vi "Text control 2 v6.9.vi"() -> ()   [LabVIEW 2016]
panel:
  in  "Tab Control":enum32{"Main", "Other parameters"}(tab)
  in  "Plot sample extrema vs time":bool
  out "Line running":i32
  out "Total lines":i32
  out "Path":path=path "C:/users/rlp38/09Apr2009LTtesting/test2.txt"
  out "I vs Vg":cluster{"Y data in":dbl[], "X data in":dbl[]}[](graph)
  out "Is max":dbl format="%.2e"
  out "Id max":dbl format="%.2e"
  out "Ig max":dbl format="%.2e"
  out "Imax vs time":cluster{"Y data in":dbl[], "X data in":dbl[]}[](graph)
  out "Imin vs time":cluster{"Y data in":dbl[], "X data in":dbl[]}[](graph)
  out "I vs Vd":cluster{"Y data in":dbl[], "X data in":dbl[]}[](graph)
  in  "Script":string="#pulsedstressV d 0.03 20 0 0.5 0.0827 5\n#\n#itime m\n#gaterangemode a\n#drainrangemode a\n#pulsed on 0.05 0 0.02\n#transfer d -10 40 1 5 40 35\n#transfer d -10 40 1 5 40 35\n#transfer d -10 40 1 5 40 35\n#output d 0 40 20 0 40 1\n#\n#\n#sample 1 0.008 221 6 0.003\n#samplei 400e-6 200 6 0.002 0.1\n#vsu2pulse -10 4\n#\n#stressV 0.016 0.03 2e-4 0.1e-3 11\n#stressI 220e-7 0.08 15\n#transfer s -1 1 0.5 -0.005 0.005 0.005\n#output s 0 0 0 -0.008 0.008 0.002"
  out "Command running:":string
  out "Serial port data":string
  out "Elapsed Time":dbl caption="Elapsed Time (s)"
  in  "Time Units":u16(ring)=1 items=["Seconds", "Minutes", "Hours"]
  in  "Time Offset":dbl caption="Set Start Time (s)"
  in  "Reset":bool
  in  "Auto Reset":bool
  in  "integration time":u32(slide) max=2 step=1 scale=0.0..2.0
  out "Is on":dbl format="%.2e"
  out "Id on":dbl format="%.2e"
  out "Ig on":dbl format="%.2e"
  out "Ion vs time":cluster{"Y data in":dbl[], "X data in":dbl[]}[](graph)
  out "Ioff vs time":cluster{"Y data in":dbl[], "X data in":dbl[]}[](graph)
  out "Ig min":dbl format="%.2e"
  out "Id min":dbl format="%.2e"
  out "Is min":dbl format="%.2e"
  out "Is off":dbl format="%.2e"
  out "Id off":dbl format="%.2e"
  out "Ig off":dbl format="%.2e"
  in  "Integration time (long)":dbl=0.32 min=0.04 max=2.0 step=0.02 format="%.2f"
  in  "Integration time (short)":dbl=0.0019 min=8e-05 max=0.0019 step=8e-05 format="%^.0e"
  in  "Drain: Compliance":dbl=0.001 format="%.8f"
  in  "Gate: Compliance":dbl=0.001 format="%.8f"
  in  "Interrupt scan":bool
  in  "Interrupt program":bool
  in  "Plot output curve extrema vs time":bool
  in  "Plot transfer curve extrema vs time":bool
  out "I vs time (Bias Stress)":cluster{"Y data in":dbl[], "X data in":dbl[]}[](graph)
  in  "Sample I - Probe 4 (Disabled)":u32(ring)=3 items=["SMU1  ", "SMU2  ", "SMU3  ", "SMU4  ", "SMU5  ", "SMU6  "]
  in  "Sample I - Source/Common":u32(ring) items=["SMU1  ", "SMU2  ", "SMU3  ", "SMU4  ", "SMU5  ", "SMU6  "]
  in  "Sample I - Probe 3 (Disabled)":u32(ring)=2 items=["SMU1  ", "SMU2  ", "SMU3  ", "SMU4  ", "SMU5  ", "SMU6  "]
  in  "Sample I - Drain/Gate":u32(ring)=1 items=["SMU1  ", "SMU2  ", "SMU3  ", "SMU4  ", "SMU5  ", "SMU6  "]
  in  "Sample - Probe 4":u32(ring)=3 items=["SMU1  ", "SMU2  ", "SMU3  ", "SMU4  ", "SMU5  ", "SMU6  "]
  in  "Sample - Source/Common":u32(ring) items=["SMU1  ", "SMU2  ", "SMU3  ", "SMU4  ", "SMU5  ", "SMU6  "]
  in  "Sample - Gate":u32(ring)=2 items=["SMU1  ", "SMU2  ", "SMU3  ", "SMU4  ", "SMU5  ", "SMU6  "]
  in  "Sample - Drain":u32(ring)=1 items=["SMU1  ", "SMU2  ", "SMU3  ", "SMU4  ", "SMU5  ", "SMU6  "]
  in  "Gate Range\nmode":u16(ring) items=["Auto", "Limited", "Fixed"]
  in  "Gate Range":u8(slide)=3 max=11 scale=0.0..11.0
  in  "Source/Drain\nRange mode":u16(ring) items=["Auto", "Limited", "Fixed"]
  in  "Source/Drain Range":u8(slide)=3 max=11 scale=0.0..11.0
  in  "Panel Controls":T1={"Emergency Stop"=refnum, "TransGraph Max"=1e-05, "Text/Graph (text=false)"=TRUE} {"TransGraph Max" format="%.2e"}
  in  "Panel Controls 2":T2={"Emergency Stop"=refnum, "TransGraph Max"=1e-05, "Text/Graph (text=false)"=TRUE, "TransGraph Min"=1e-11} {"TransGraph Min" format="%.2e"; "TransGraph Max" format="%.2e"}
  out "error out":errorcluster
  in  "Delay before read (ms)":u32=1000
  in  "byte count":u32=64
  in  "Serial End Mode for Reads":u16(ring)=2 items=["None", "LastBit", "TermChar"]
  in  "Timeout (ms)":u32=10000
  in  "Enable Termination\nChar (T)":bool=TRUE
  in  "Termination char\n(0xA = '\\n' = LF)\n(0xD = '\\r' = CR)":u8=13 format="%.0x"
  in  "flow control":u16(ring) items=["None"=0, "XON/XOFF"=1, "RTS/CTS"=2, "DTR/DSR"=4]
  in  "stop bits":u16(ring)=10 items=["1.0"=10, "1.5"=15, "2.0"=20]
  in  "parity":u16(ring) items=["None", "Odd", "Even", "Mark", "Space"]
  in  "data bits":u16=8 min=5 max=8 step=1
  in  "VISA resource name":refnum<visa-resource-name>="COM6"
  in  "baud rate":u32=9600
  out "Timings Indicator":T3
  in  "Timings (overwritten by the Front Panel)":T4={"integration time"=0, "Short/Long integration time"=0.00064, "hold time (sec)"=0.0, "delay time (sec)"=0.0, "Step Time (0 disables)"=0.0, "sweep method"=0, "Pulse period"=0.005, "Base voltage"=0.0, "Pulse width"=0.0005} {"Pulse width" min=0.0005 max=0.1 step=0.0001 format="%.4f"; "Base voltage" format="%^.4e"; "Pulse period" min=0.005 max=1.0 step=0.0001 format="%.4f"; "sweep method" items=["Continuous", "Pulsed"]; "Step Time (0 disables)" format="%.2f"; "delay time (sec)" format="%.4f"; "hold time (sec)" format="%.4f"; "Short/Long integration time" format="%^.0e"; "integration time" scale=0.0..2.0}
  in  "Probe 4":cluster{"on/off":bool, "Voltage":dbl} {"Voltage" min=-100.0 max=100.0 format="%.2f"}
  in  "Full Reset":bool
  in  "Standby":T5
  out "Probe 4 Indicator":cluster{"on/off":bool, "Voltage":dbl} {"Voltage" min=-100.0 max=100.0 format="%.2f"}
  in  "Transfer/Output - Drain":u32(ring)=1 items=["SMU1  ", "SMU2  ", "SMU3  ", "SMU4  ", "SMU5  ", "SMU6  "]
  in  "Transfer/Output - Gate":u32(ring)=2 items=["SMU1  ", "SMU2  ", "SMU3  ", "SMU4  ", "SMU5  ", "SMU6  "]
  in  "Transfer/Output - Source/Common":u32(ring) items=["SMU1  ", "SMU2  ", "SMU3  ", "SMU4  ", "SMU5  ", "SMU6  "]
  in  "Transfer/Output - Probe 4":u32(ring)=3 items=["SMU1  ", "SMU2  ", "SMU3  ", "SMU4  ", "SMU5  ", "SMU6  "]
  in  "Pulsed Stress V - Probe 4":u32(ring)=3 items=["SMU1  ", "SMU2  ", "SMU3  ", "SMU4  ", "SMU5  ", "SMU6  "]
  in  "Pulsed Stress V - Vextra":u32(ring)=1 items=["VSU1  ", "VSU2  "]
  in  "Pulsed Stress V - Drain":u32(ring)=1 items=["SMU1  ", "SMU2  ", "SMU3  ", "SMU4  ", "SMU5  ", "SMU6  "]
  in  "Pulsed Stress V - Source/Common":u32(ring) items=["SMU1  ", "SMU2  ", "SMU3  ", "SMU4  ", "SMU5  ", "SMU6  "]
  in  "Pulsed Stress V - Gate":u32(ring)=2 items=["SMU1  ", "SMU2  ", "SMU3  ", "SMU4  ", "SMU5  ", "SMU6  "]
  in  "FPP - Drain":u32(ring)=1 items=["SMU1  ", "SMU2  ", "SMU3  ", "SMU4  ", "SMU5  ", "SMU6  "]
  in  "FPP - Gate":u32(ring)=2 items=["SMU1  ", "SMU2  ", "SMU3  ", "SMU4  ", "SMU5  ", "SMU6  "]
  in  "FPP - Probe 1":u32(ring) items=["SMU1  ", "SMU2  ", "SMU3  ", "SMU4  ", "SMU5  ", "SMU6  "]
  in  "FPP - Probe 2":u32(ring)=3 items=["SMU1  ", "SMU2  ", "SMU3  ", "SMU4  ", "SMU5  ", "SMU6  "]
  in  "FPP - Source":u32(ring) items=["VSU1  ", "VSU2  "]
  in  "Stress V - Drain":u32(ring)=1 items=["SMU1  ", "SMU2  ", "SMU3  ", "SMU4  ", "SMU5  ", "SMU6  "]
  in  "Stress V - Gate":u32(ring)=2 items=["SMU1  ", "SMU2  ", "SMU3  ", "SMU4  ", "SMU5  ", "SMU6  "]
  in  "Stress V - Source/Common":u32(ring) items=["SMU1  ", "SMU2  ", "SMU3  ", "SMU4  ", "SMU5  ", "SMU6  "]
  in  "Stress I - Drain/Gate":u32(ring)=1 items=["SMU1  ", "SMU2  ", "SMU3  ", "SMU4  ", "SMU5  ", "SMU6  "]
  in  "Stress I - Source/Common":u32(ring) items=["SMU1  ", "SMU2  ", "SMU3  ", "SMU4  ", "SMU5  ", "SMU6  "]
  in  "VSU2 Stress - Source/Common":u32(ring) items=["SMU1  ", "SMU2  ", "SMU3  ", "SMU4  ", "SMU5  ", "SMU6  "]
  in  "VISA resource name in":refnum<visa-resource-name>="GPIB0::14::INSTR"
  in  "Gate":T6={"Gate Start"=0.0, "Gate Stop"=2.0, "Gate Step (linear only)"=1.0, "Gate Compliance"=0.0001, "Gate PComp"=0.0, "Range mode"=0, "Range"=6} {"Range" max=11 scale=0.0..11.0; "Range mode" items=["Auto", "Limited", "Fixed"]; "Gate PComp" format="%^.2e"; "Gate Compliance" format="%^.2e"; "Gate Step (linear only)" format="%^.4e"; "Gate Stop" format="%^.4e"; "Gate Start" format="%^.4e"}
  in  "Drain 2":T7={"Drain Start"=0.0, "Drain Stop"=2.0, "Drain Compliance"=0.0001, "Drain Step"=1.0, "Drain PComp"=0.0, "Range mode"=0, "Range"=6} {"Range" max=11 scale=0.0..11.0; "Range mode" items=["Auto", "Limited", "Fixed"]; "Drain PComp" format="%^.2e"; "Drain Step" format="%^.4e"; "Drain Compliance" format="%^.2e"; "Drain Stop" format="%^.4e"; "Drain Start" format="%^.4e"}
  # "Time"
  # "Syntax:\nitime [s|m|l] time(sec): [s|m|l] determines the integration time setting (small|medium|long) and time sets the value.\nNOTE: The value of the integration time has to be within the range allowed by its category (s|m|l), otherwise, the closest value will be used. (e.g. if the category is set to short but the time value is very long, the actual value used will be the maximum short integration time.\nIntegration times:\n    Short: Default: 640 us. Range: 8E-5 - 1.92E-3 seconds.\n    Medium: Fixed at 1 NPL cycle (0.02 seconds).\n    Long: Default: 16 NPL cycles (0.32 seconds). Range: 2-100 NPL cycles (0.04 seconds - 2 seconds).\ngaterangemode [a|l|f]\ndrainrangemode [a|l|f]\npulsed [on|off] PulsePeriod(sec) PulseBaseVoltage PulseONWidth(sec)\nstandby [on l off]\nwait NumMilliseconds\nwait-min NumMinutes\n# texthere = comment\nProbe4 [ON|OFF] Voltage\ntransfer [s|d] VgStart VgStop VgStep VdStart VdStop VdStep\noutput [s|d] VgStart VgStop VgStep VdStart VdStop VdStep\nsample Vg Vd NumSamples Time(s) SampleInterval(s)\nsamplei Idg NumSamples Time(s) SampleInterval(s) VDGcompliance\n100 samples is approximately 13 seconds with medium integration\n# if in doubt use SampleInterval(s) = 0.004\n    NOTE: When doing bias stress measurements, set the Time Units to \"Seconds\", as the \"sample\" command has been configured to give the output to seconds.\nstressV VG VD IGcompliance IDcompliance Duration(sec)\nstressI IDG VDGcompliance Duration(sec)\nvsu2pulse Bias Duration(s)\npulsedstressV [s|d] VEstop VgON VgOFF Period(s) PulseONwidth(s) Vd\nsample-fpp Vg Vd NumSamples Time\nresample-fpp Vg Vd\ntransfer-fpp [s|d] VgStart VgStop VgStep VdStart VdStop VdStep\noutput-fpp [s|d] VgStart VgStop VgStep VdStart VdStop VdStep\nserial SerialPortCommand"
  # "1\n2\n3\n4\n5\n6\n7\n8\n9\n10\n11\n12\n13\n14\n15\n16\n17\n18\n19\n20"
  # "SMUs"
  # "Serial port settings"
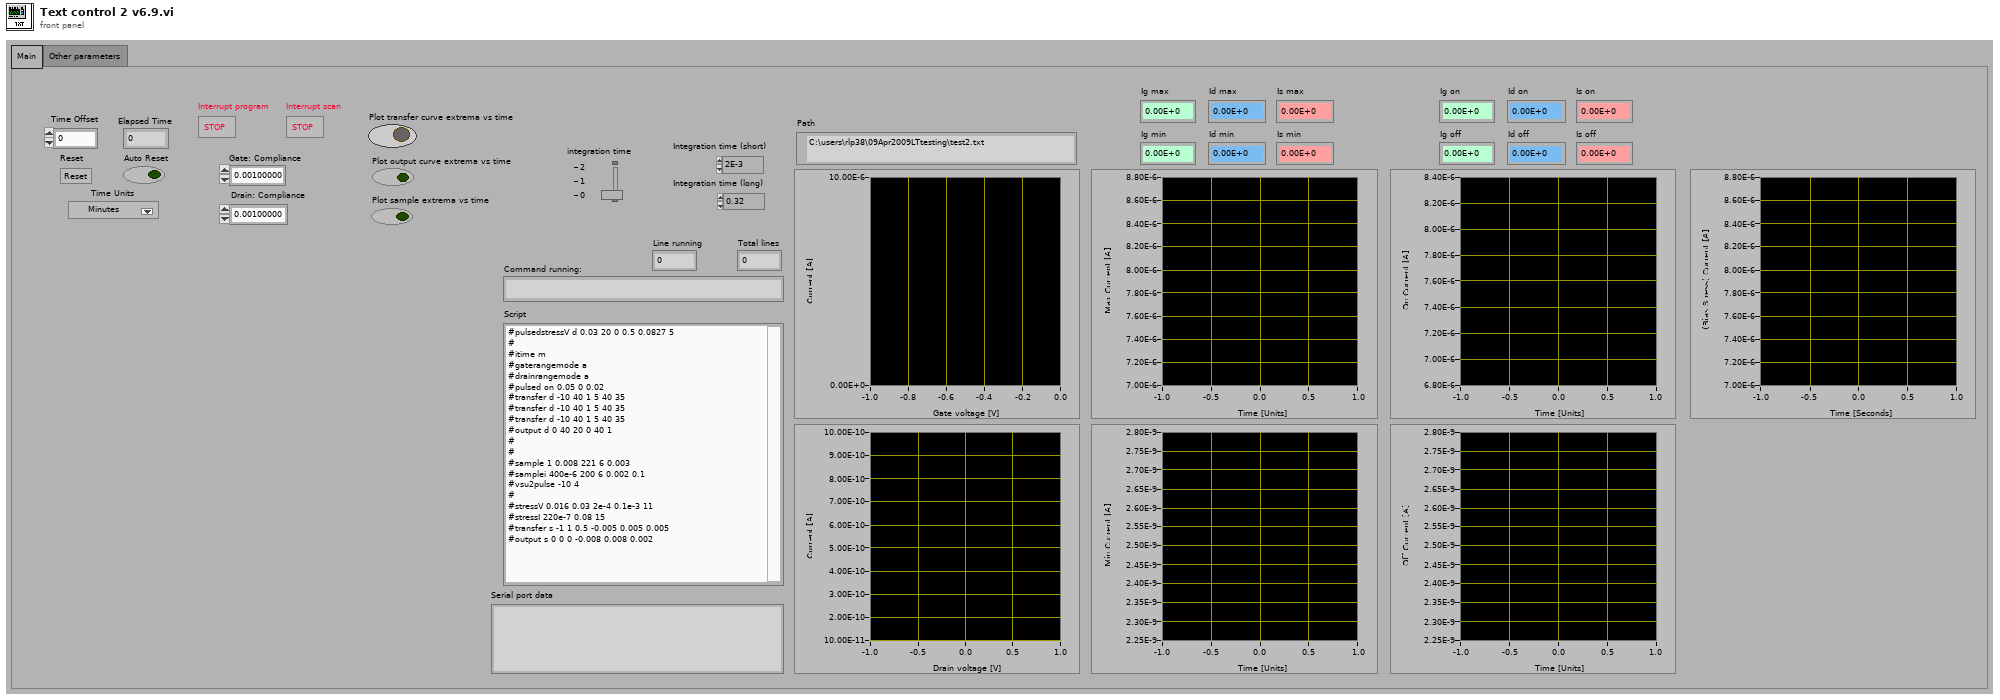
[diagram p1: front panel]
types:
  T1 = cluster{"Emergency Stop":refnum<vi>, "TransGraph Max":dbl, "Text/Graph (text=false)":bool}
  T2 = cluster{"Emergency Stop":refnum<vi>, "TransGraph Max":dbl, "Text/Graph (text=false)":bool, "TransGraph Min":dbl}
  T3 = cluster{"integration time (0:s, 1:m, 2:l)":u32, "Short/Long integration time":dbl, "hold time (sec)":dbl, "delay time (sec)":dbl, "Step Time (0 disables)":dbl, "sweep method":u16, "Pulse period":dbl, "Base voltage":dbl, "Pulse width":dbl}
  T4 = cluster{"integration time":u32, "Short/Long integration time":dbl, "hold time (sec)":dbl, "delay time (sec)":dbl, "Step Time (0 disables)":dbl, "sweep method":u16, "Pulse period":dbl, "Base voltage":dbl, "Pulse width":dbl}
  T5 = cluster{"Gate Standby":bool, "Drain Standby":bool}
  T6 = cluster{"Gate Start":dbl, "Gate Stop":dbl, "Gate Step (linear only)":dbl, "Gate Compliance":dbl, "Gate PComp":dbl, "Range mode":u16, "Range":u8}
  T7 = cluster{"Drain Start":dbl, "Drain Stop":dbl, "Drain Compliance":dbl, "Drain Step":dbl, "Drain PComp":dbl, "Range mode":u16, "Range":u8}
  T8 = enum16{"open", "replace", "create", "open or create", "replace or create", "replace or create with confirmation"}
  T9 = cluster{"V2 Start":dbl, "V2 Step":dbl, "Number of points":i32}
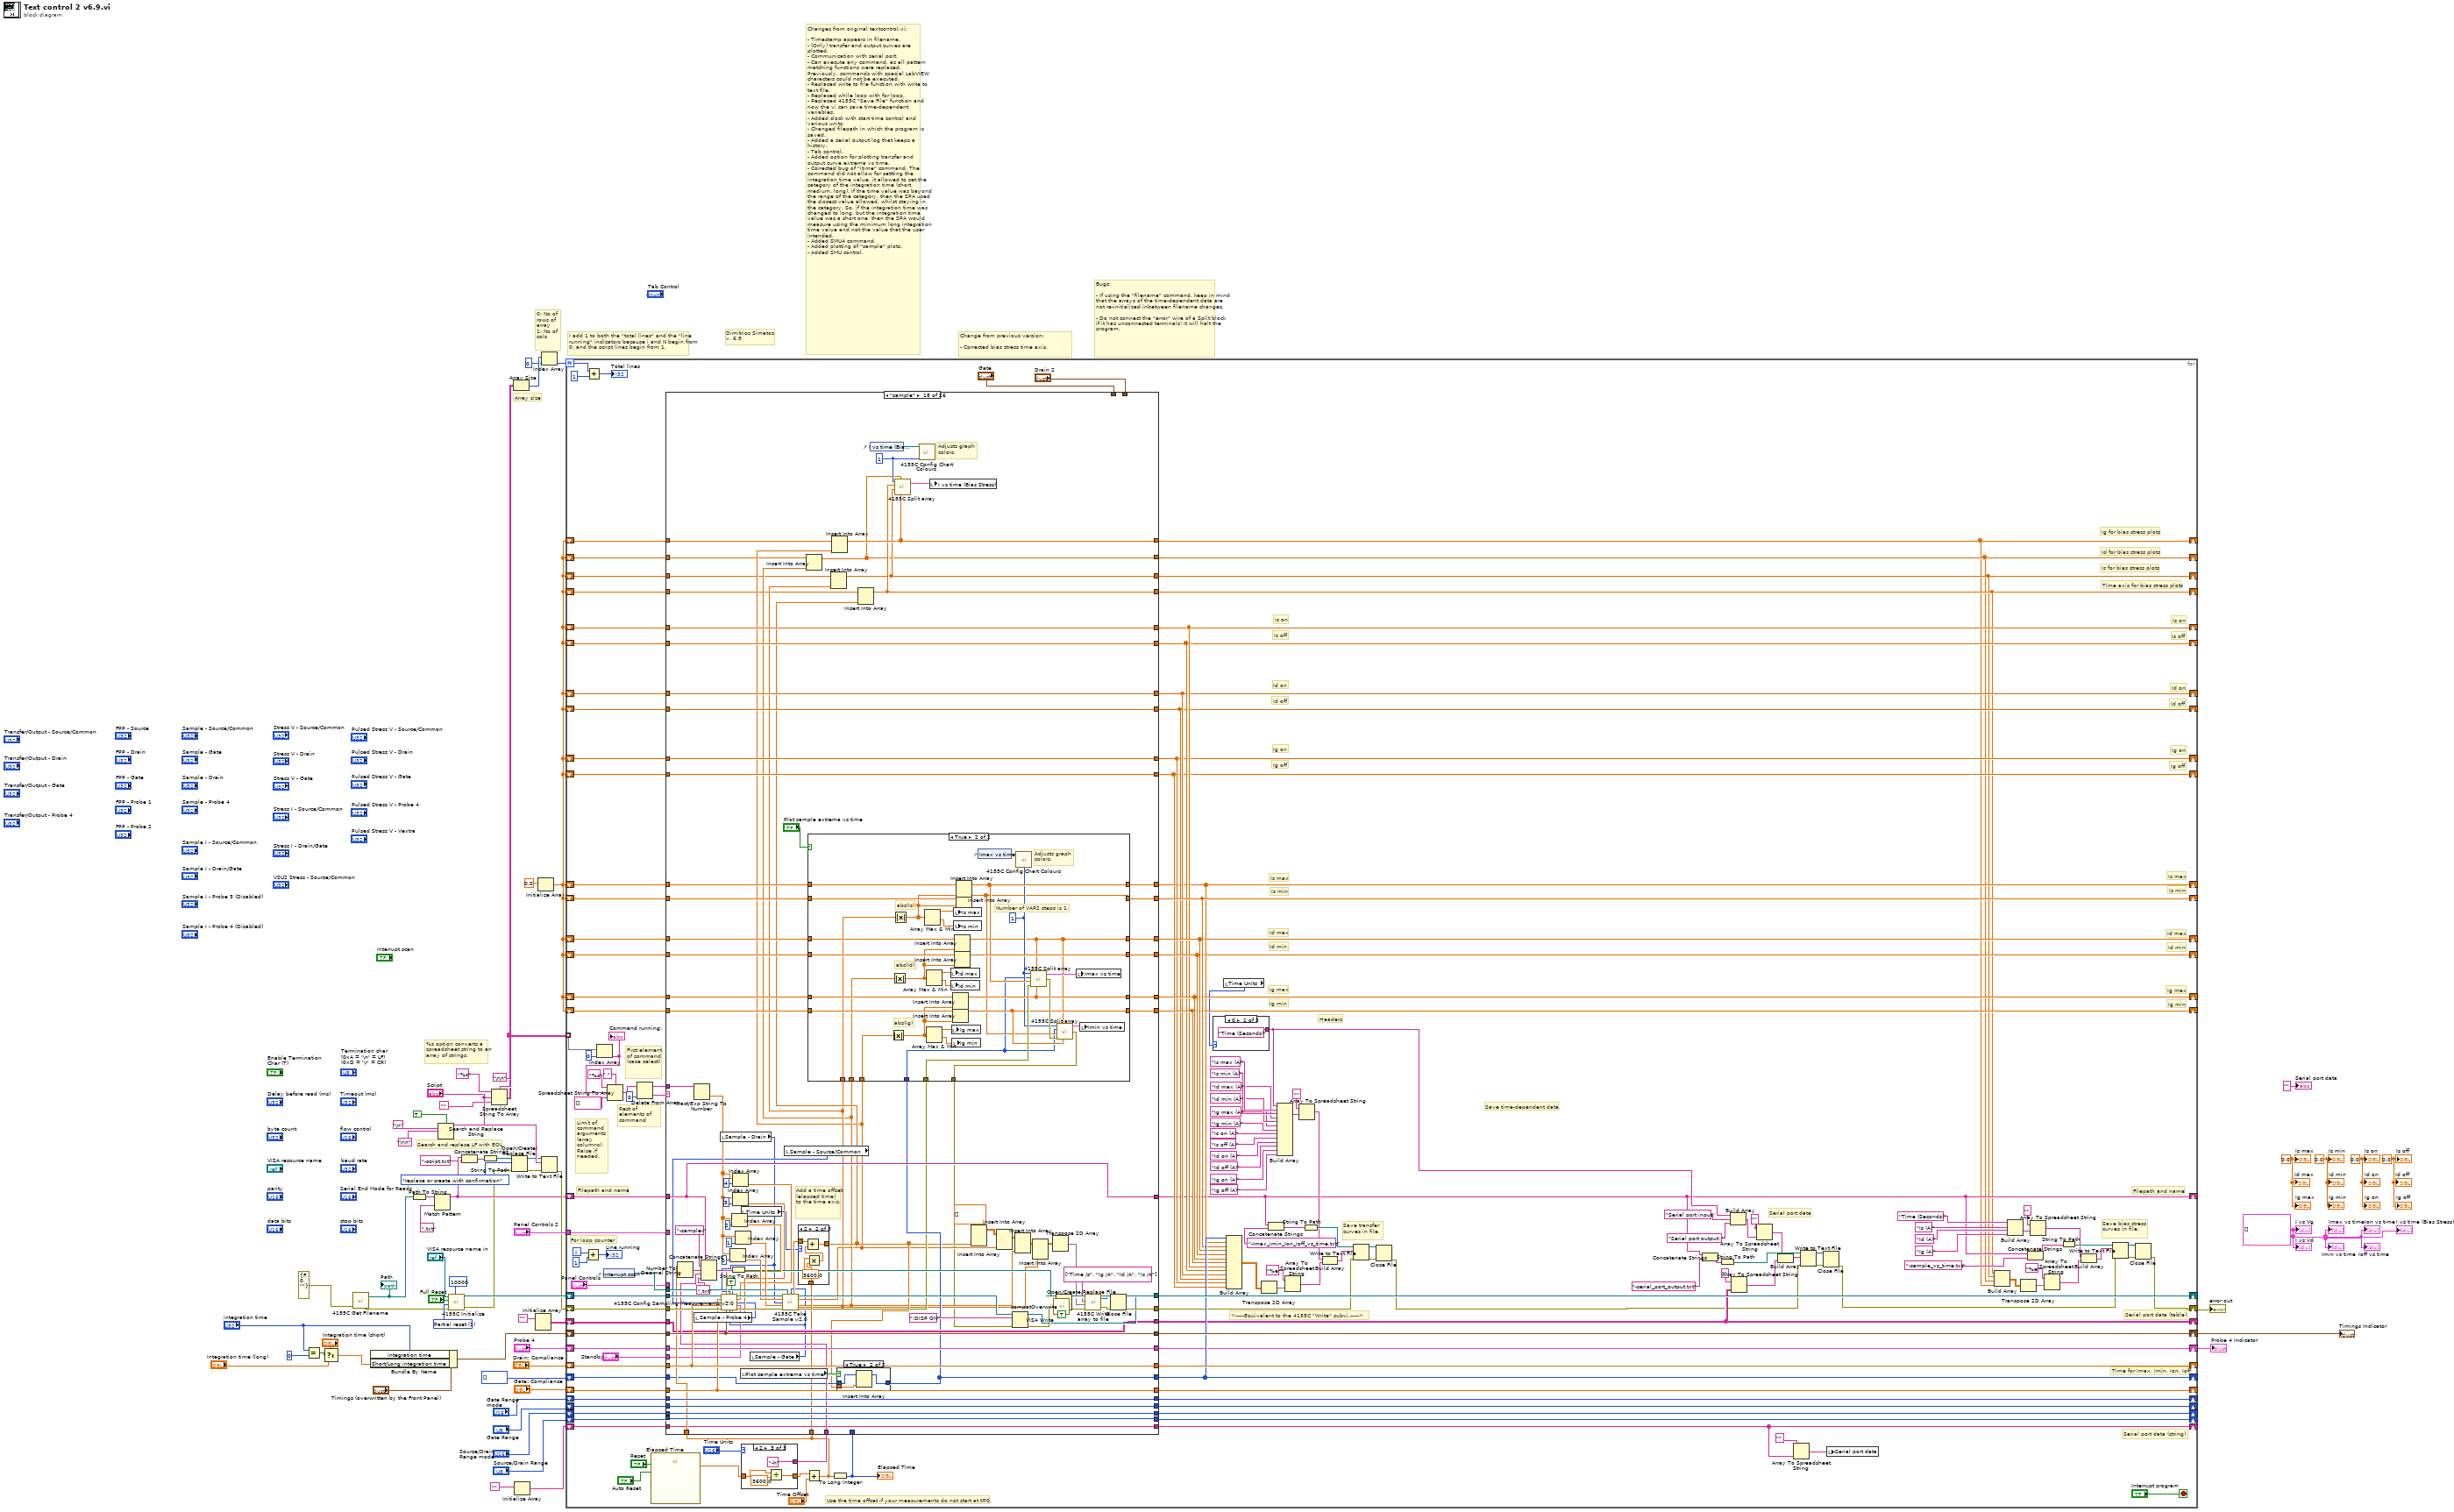
[diagram p0: block diagram]
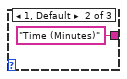
[diagram p2: hidden frame]
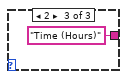
[diagram p3: hidden frame]
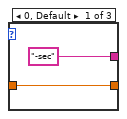
[diagram p4: hidden frame]
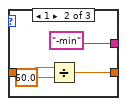
[diagram p5: hidden frame]
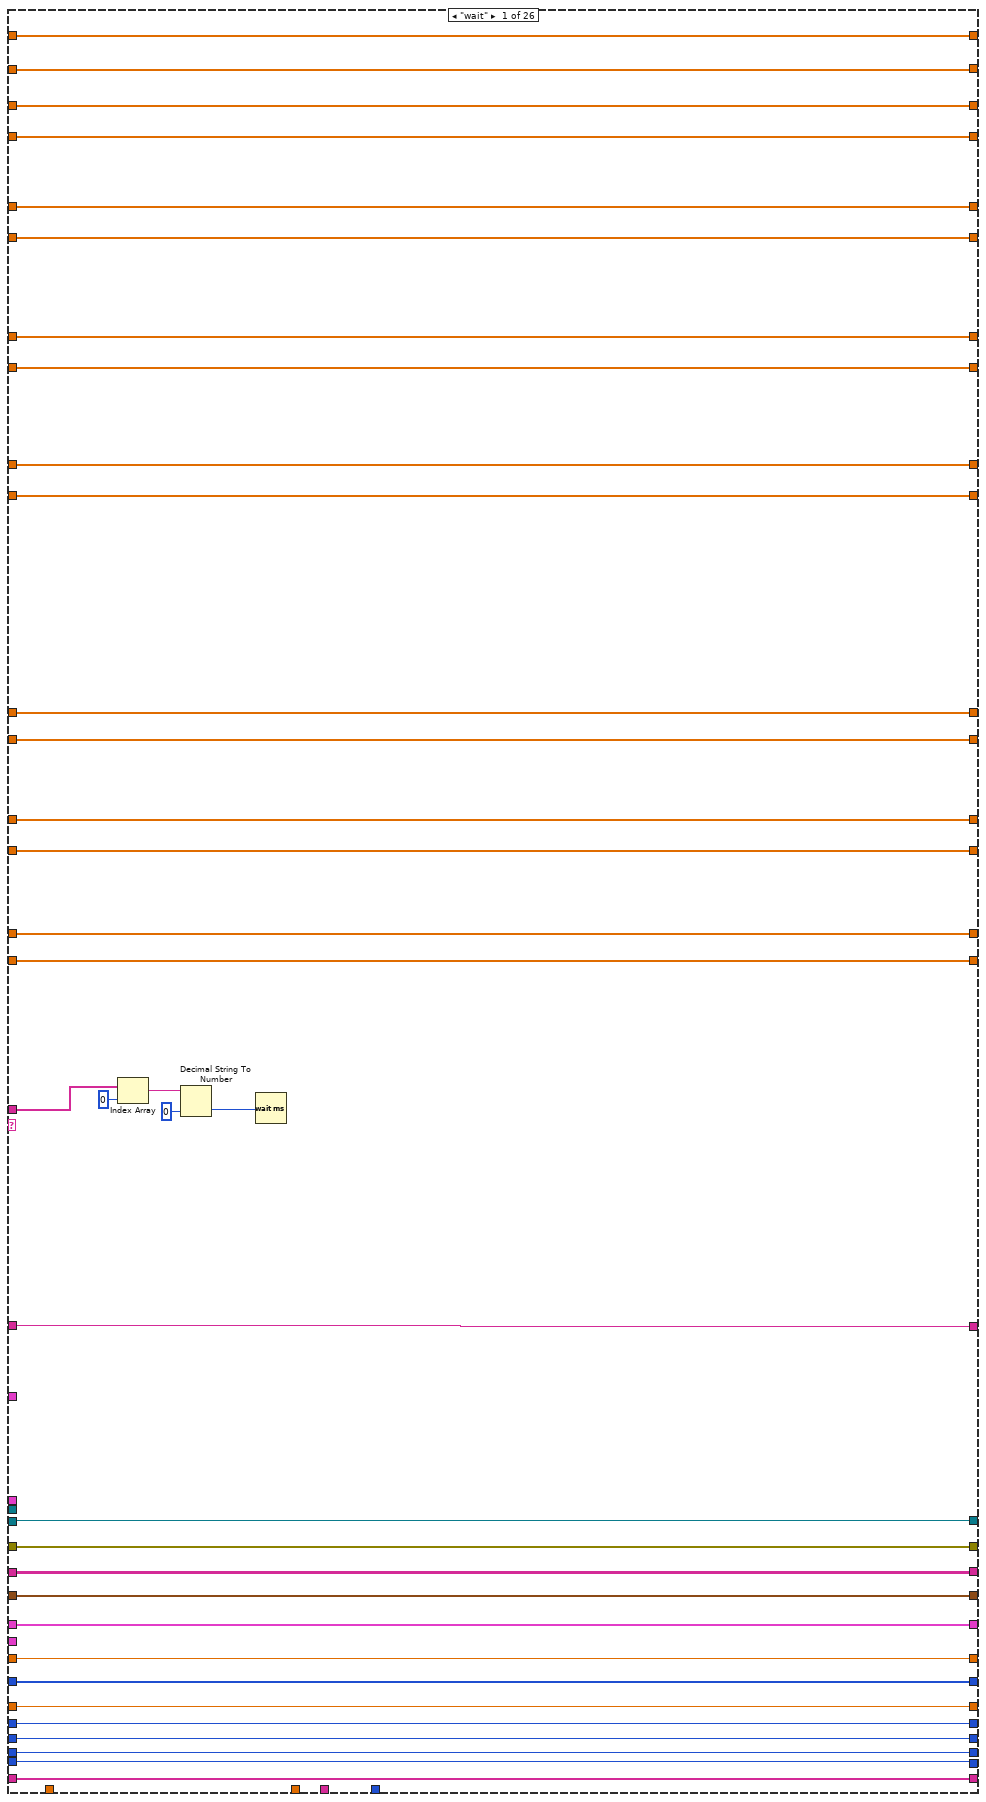
[diagram p6: hidden frame]
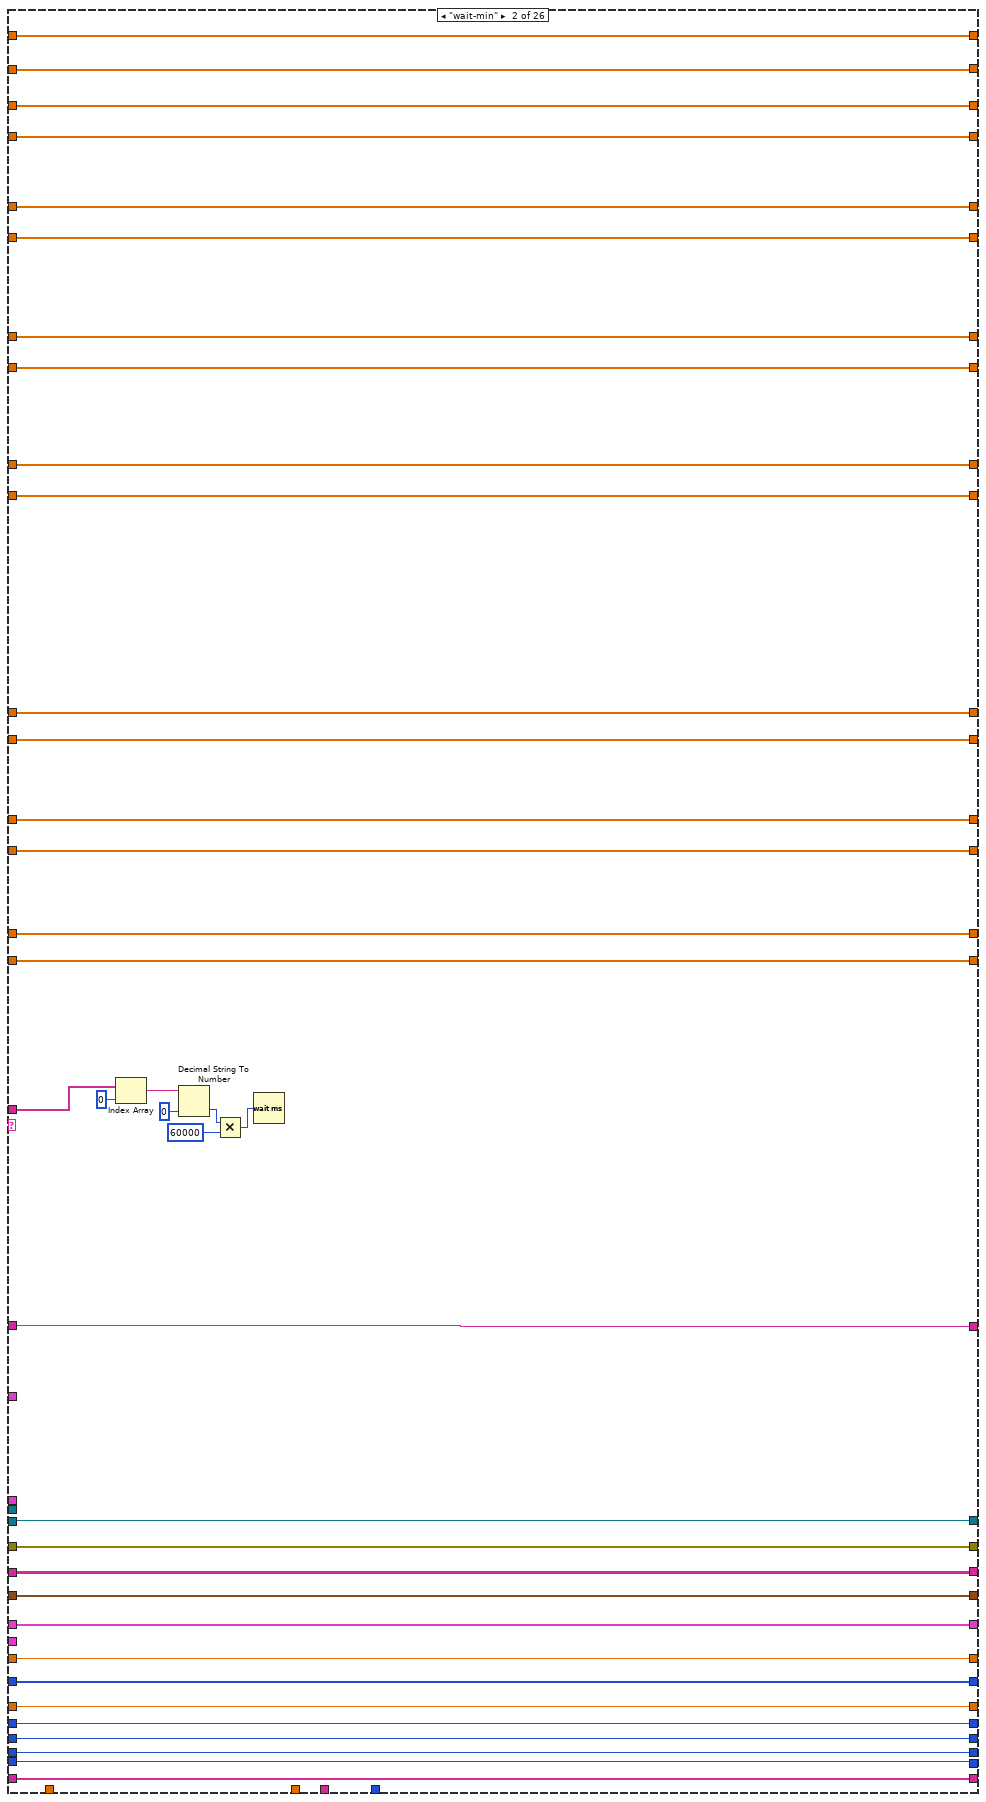
[diagram p7: hidden frame]
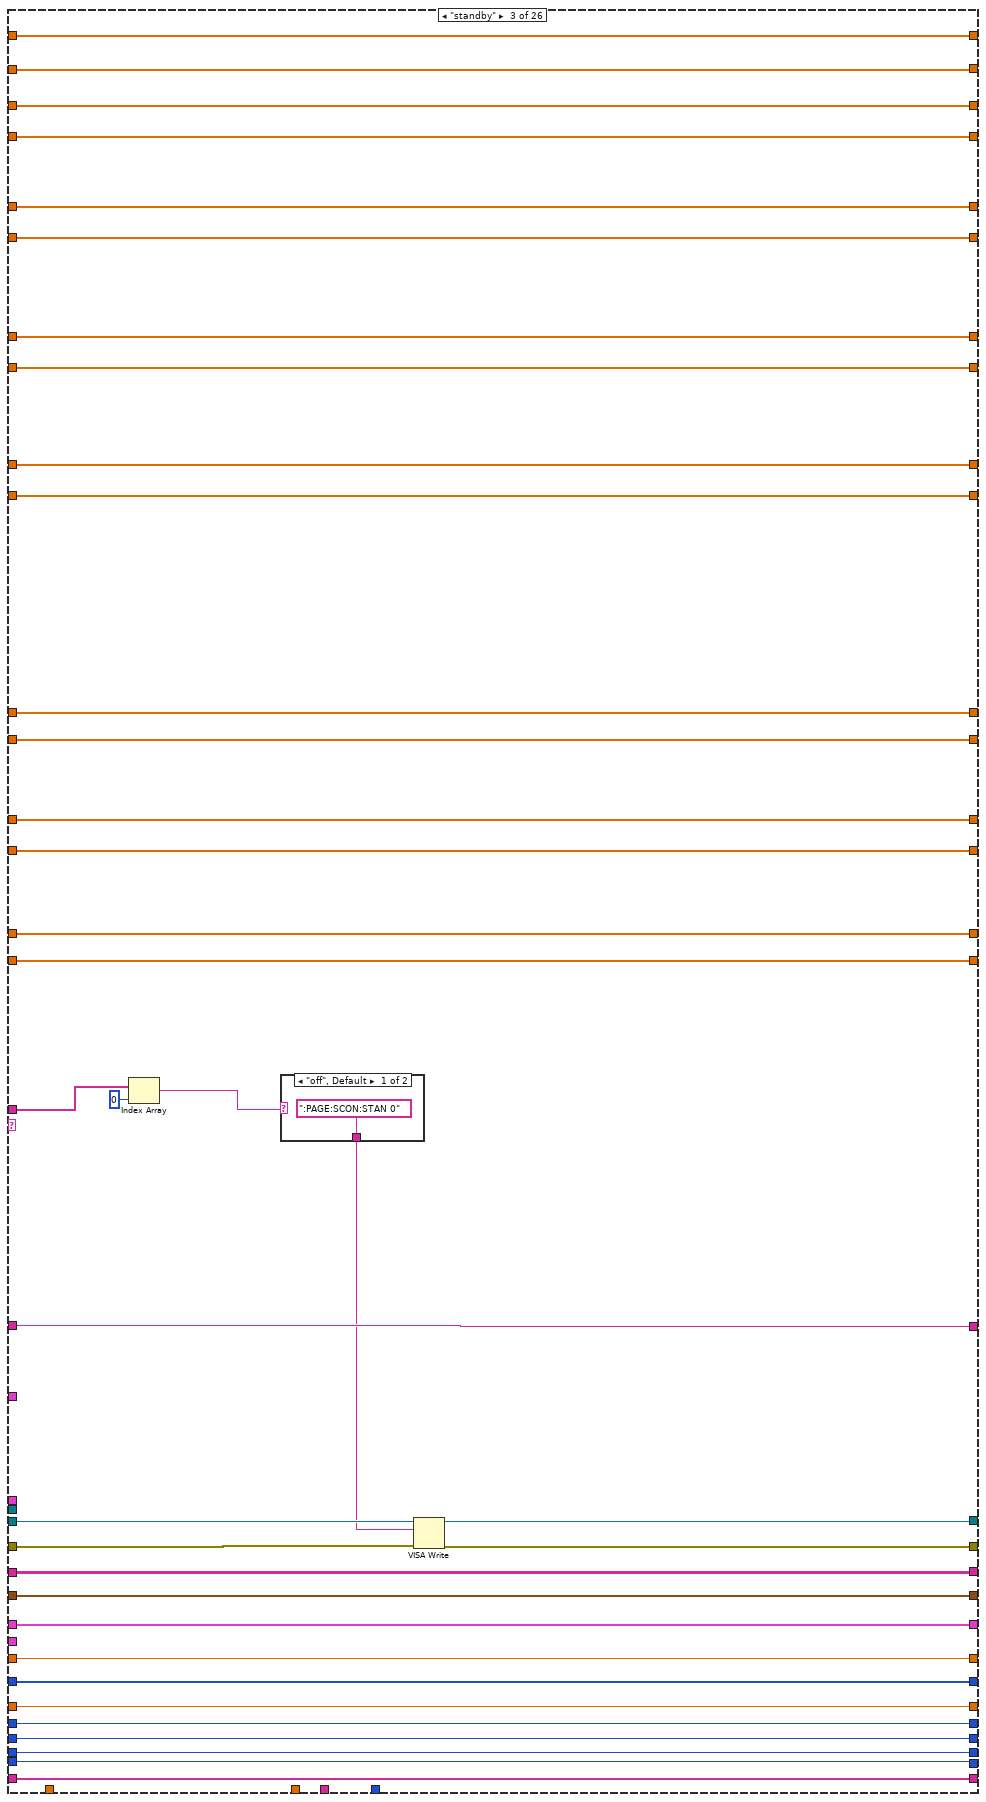
[diagram p8: hidden frame]
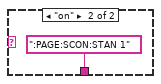
[diagram p9: hidden frame]
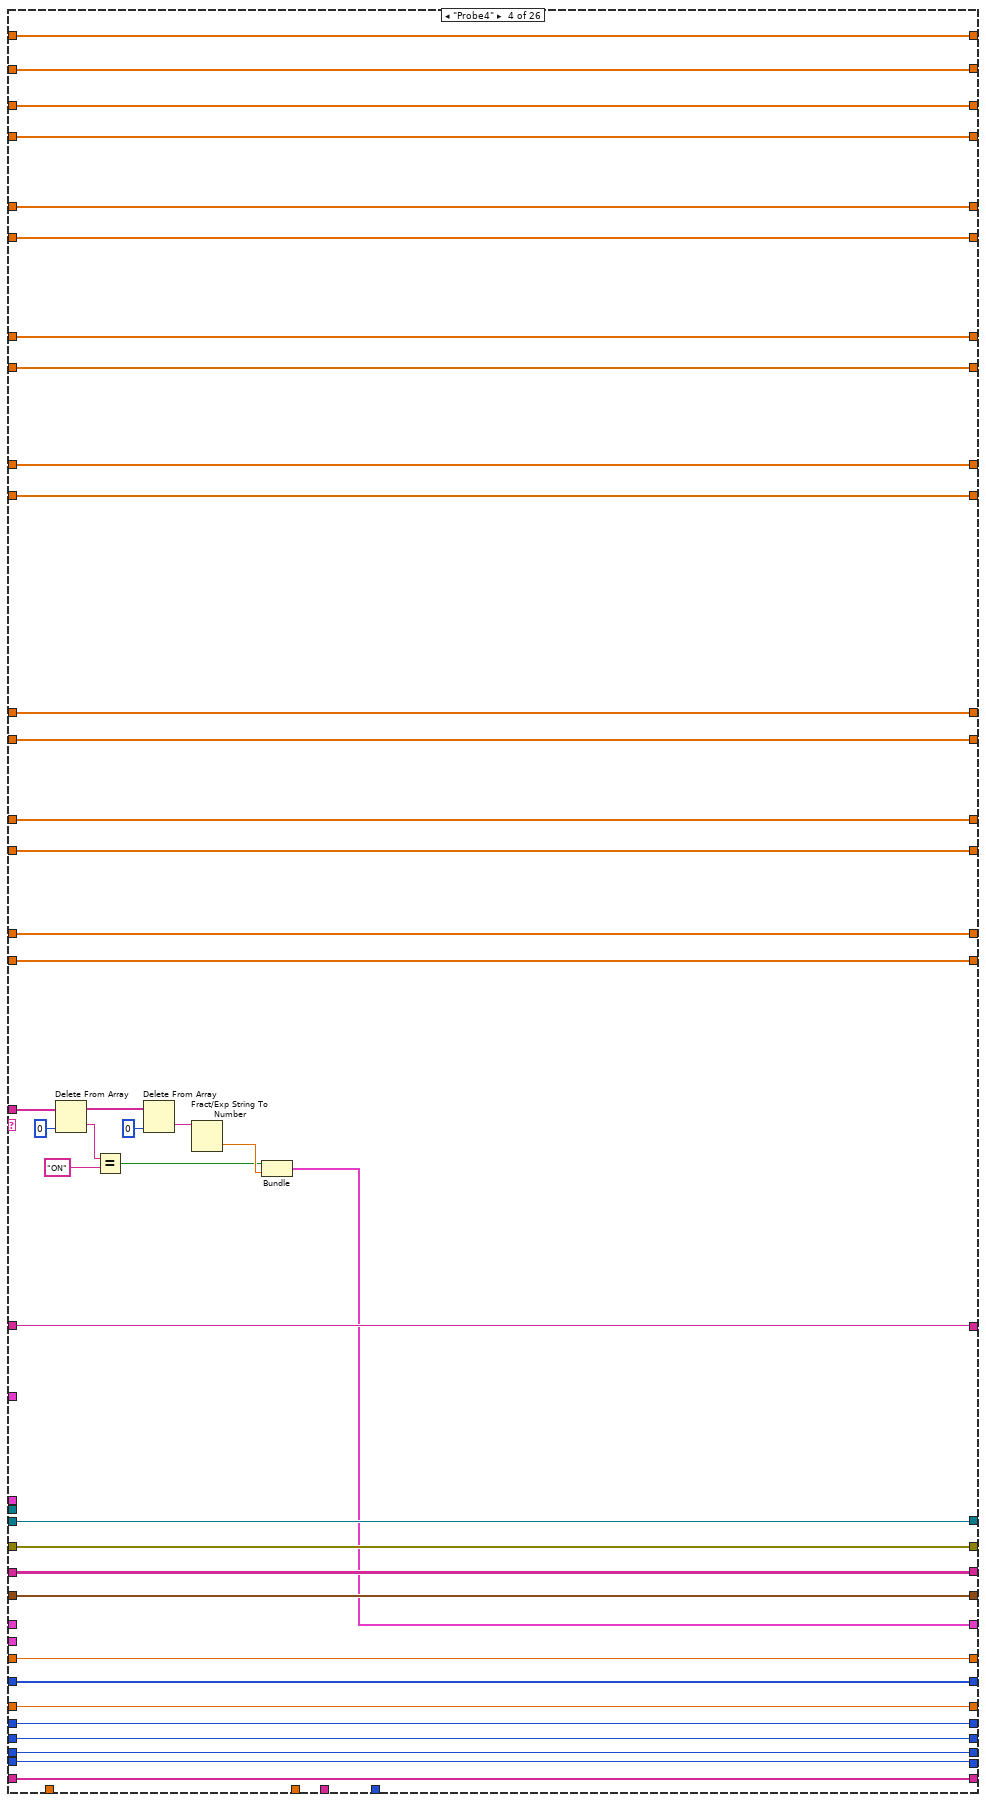
[diagram p10: hidden frame]
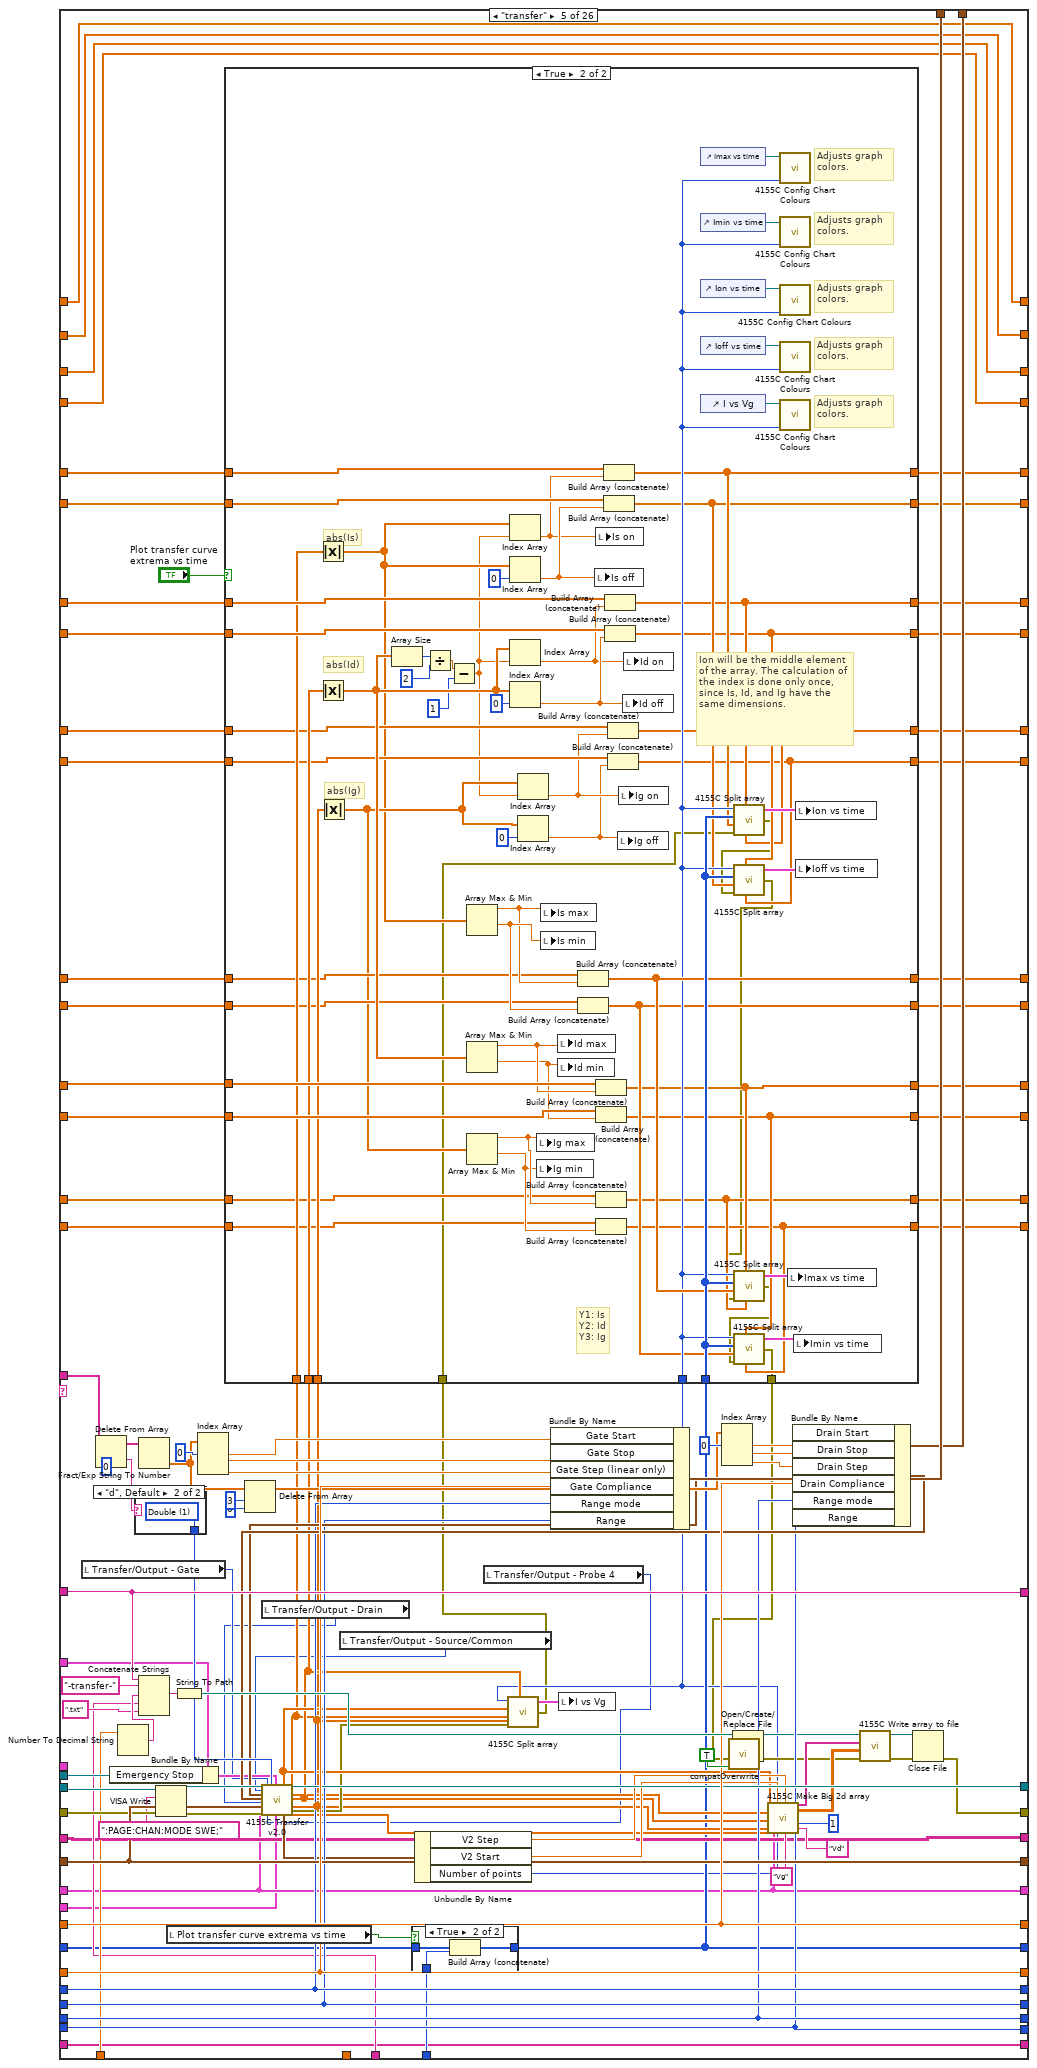
[diagram p11: hidden frame]
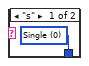
[diagram p14: hidden frame]
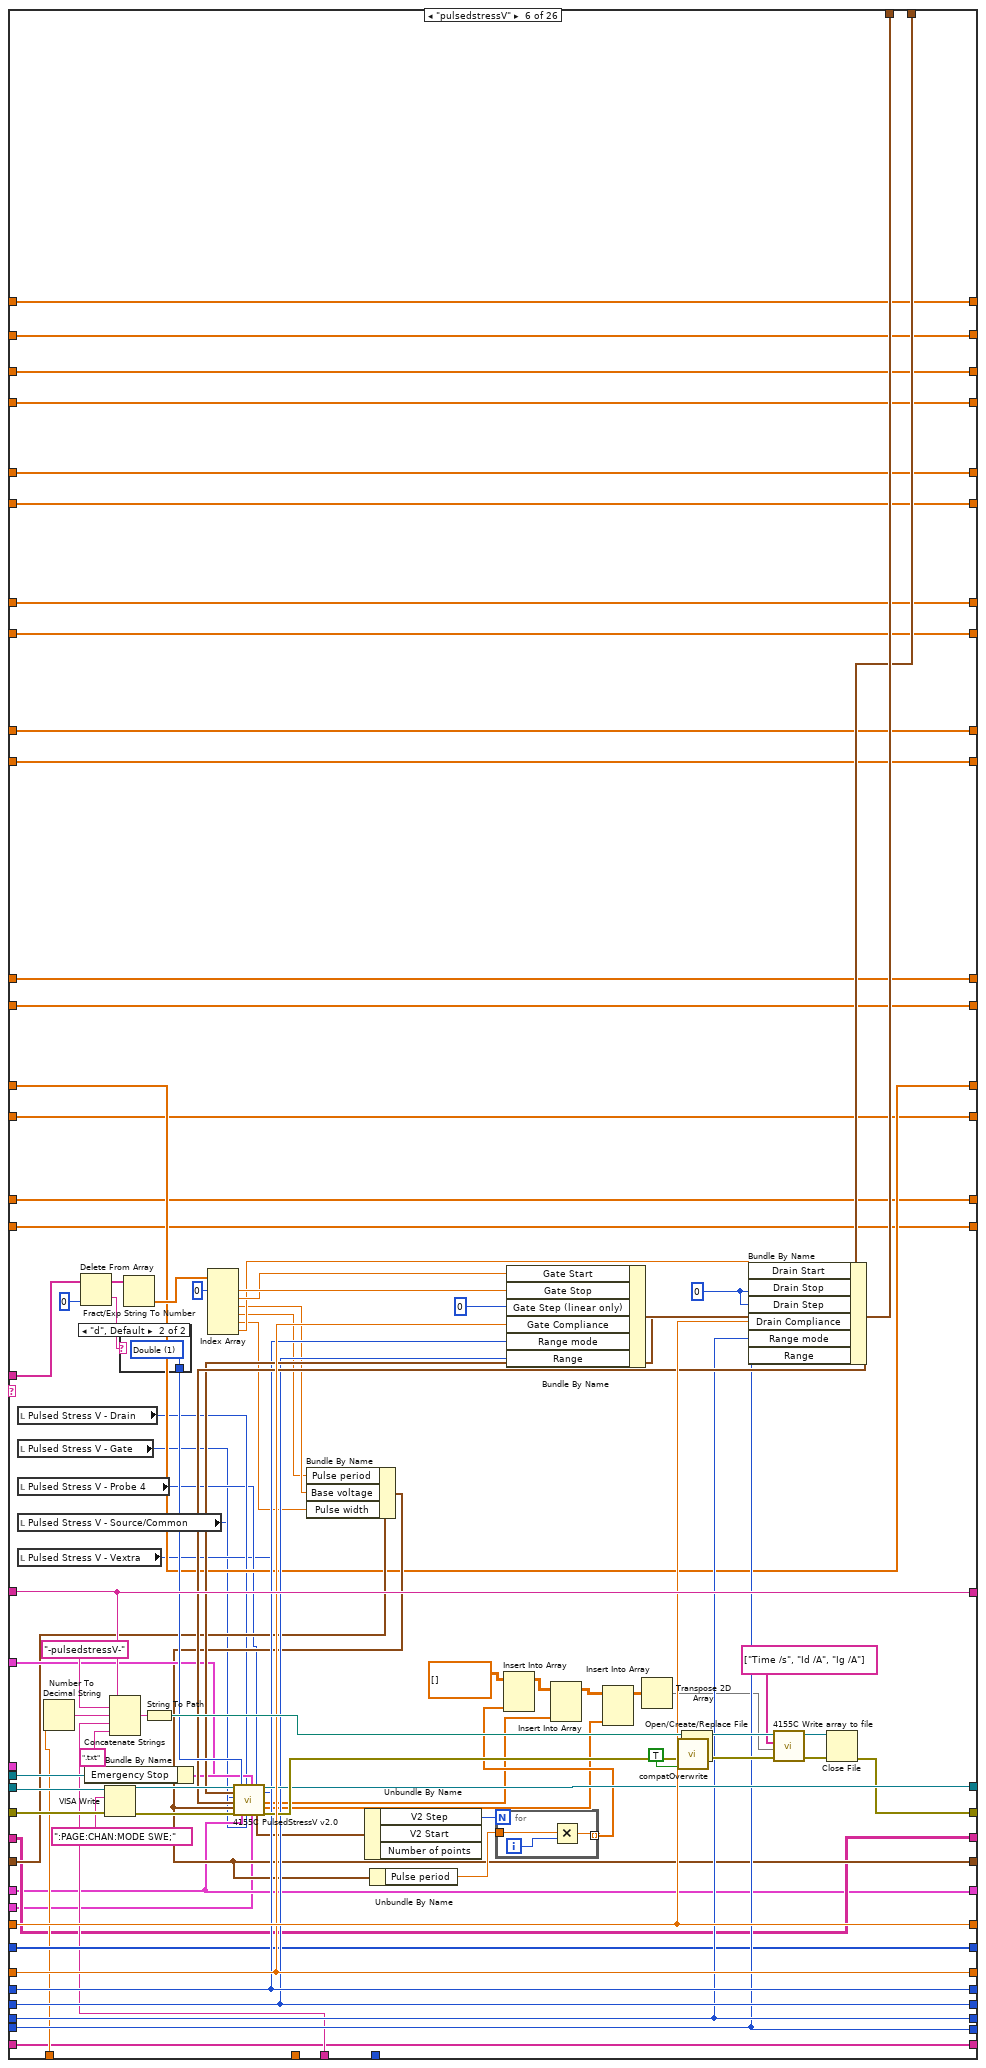
[diagram p15: hidden frame]
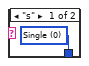
[diagram p16: hidden frame]
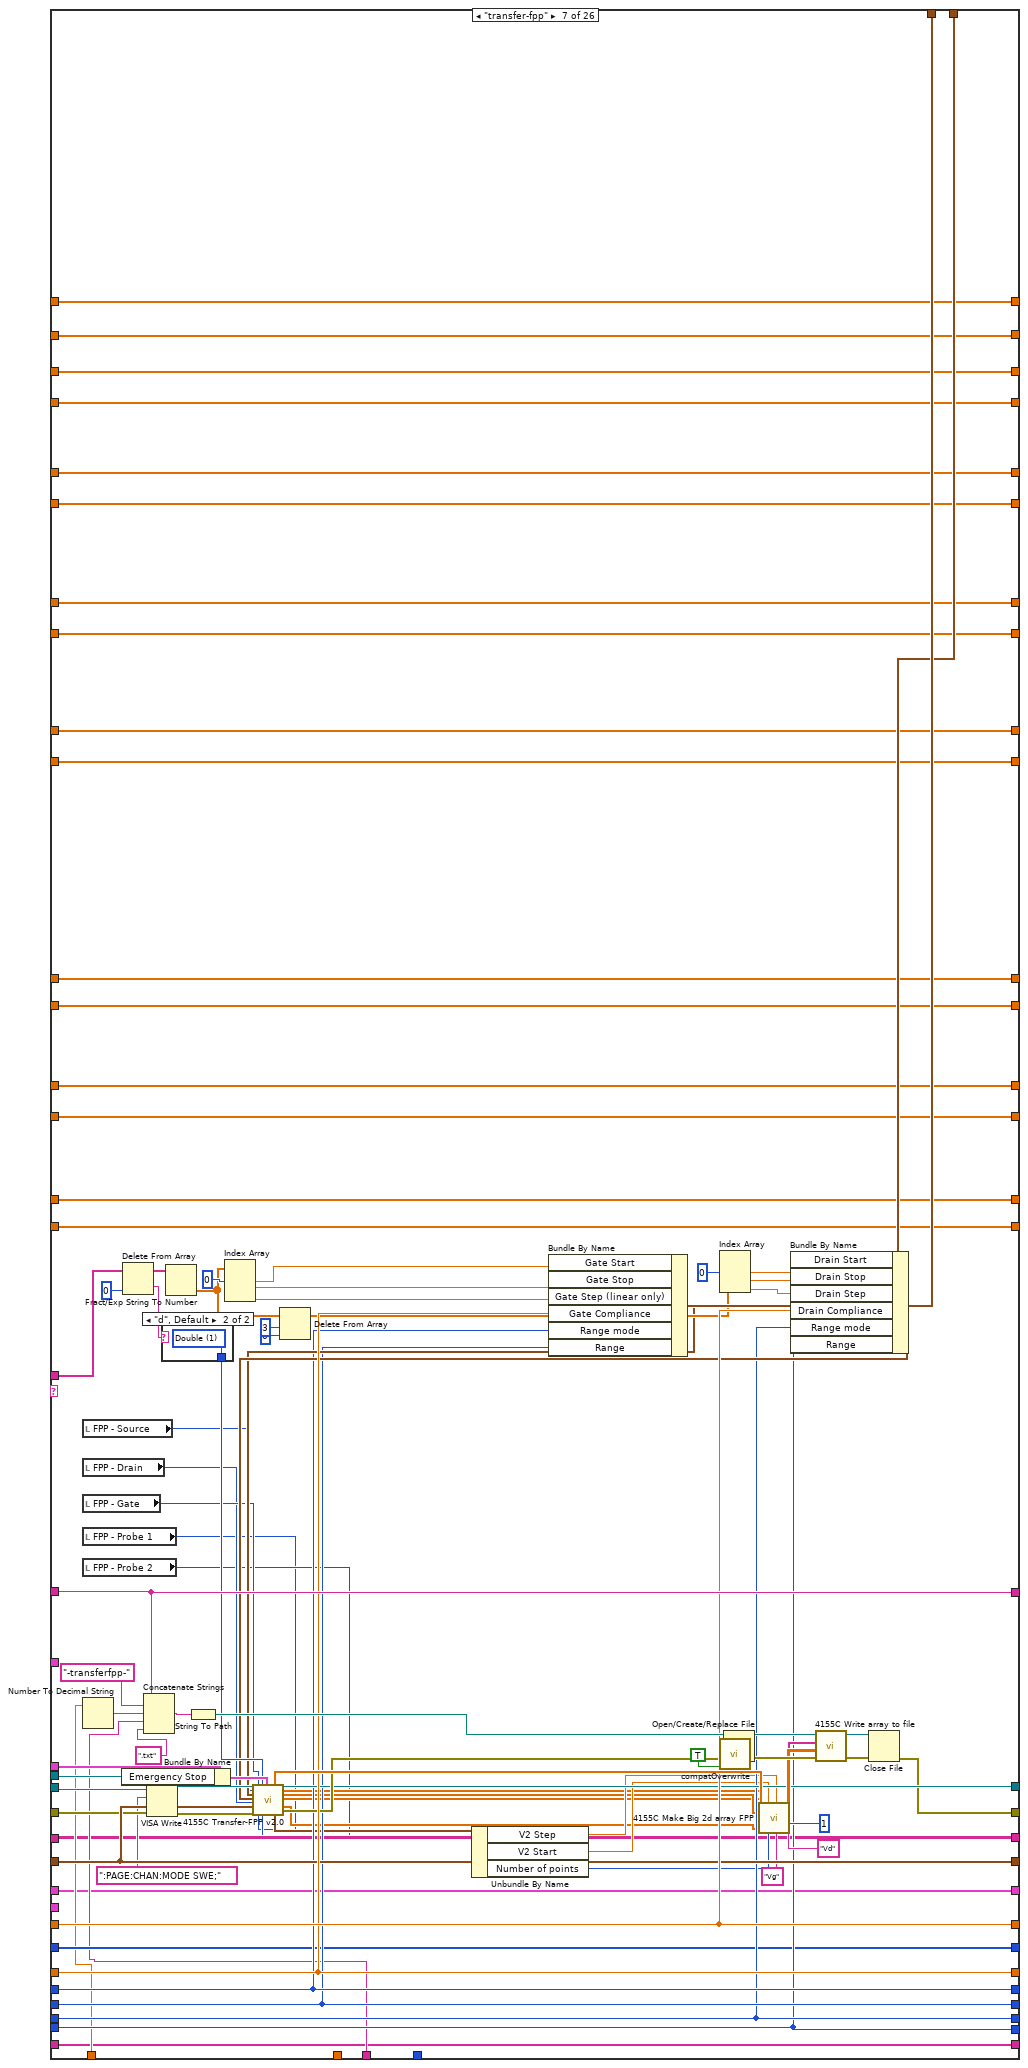
[diagram p17: hidden frame]
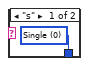
[diagram p18: hidden frame]
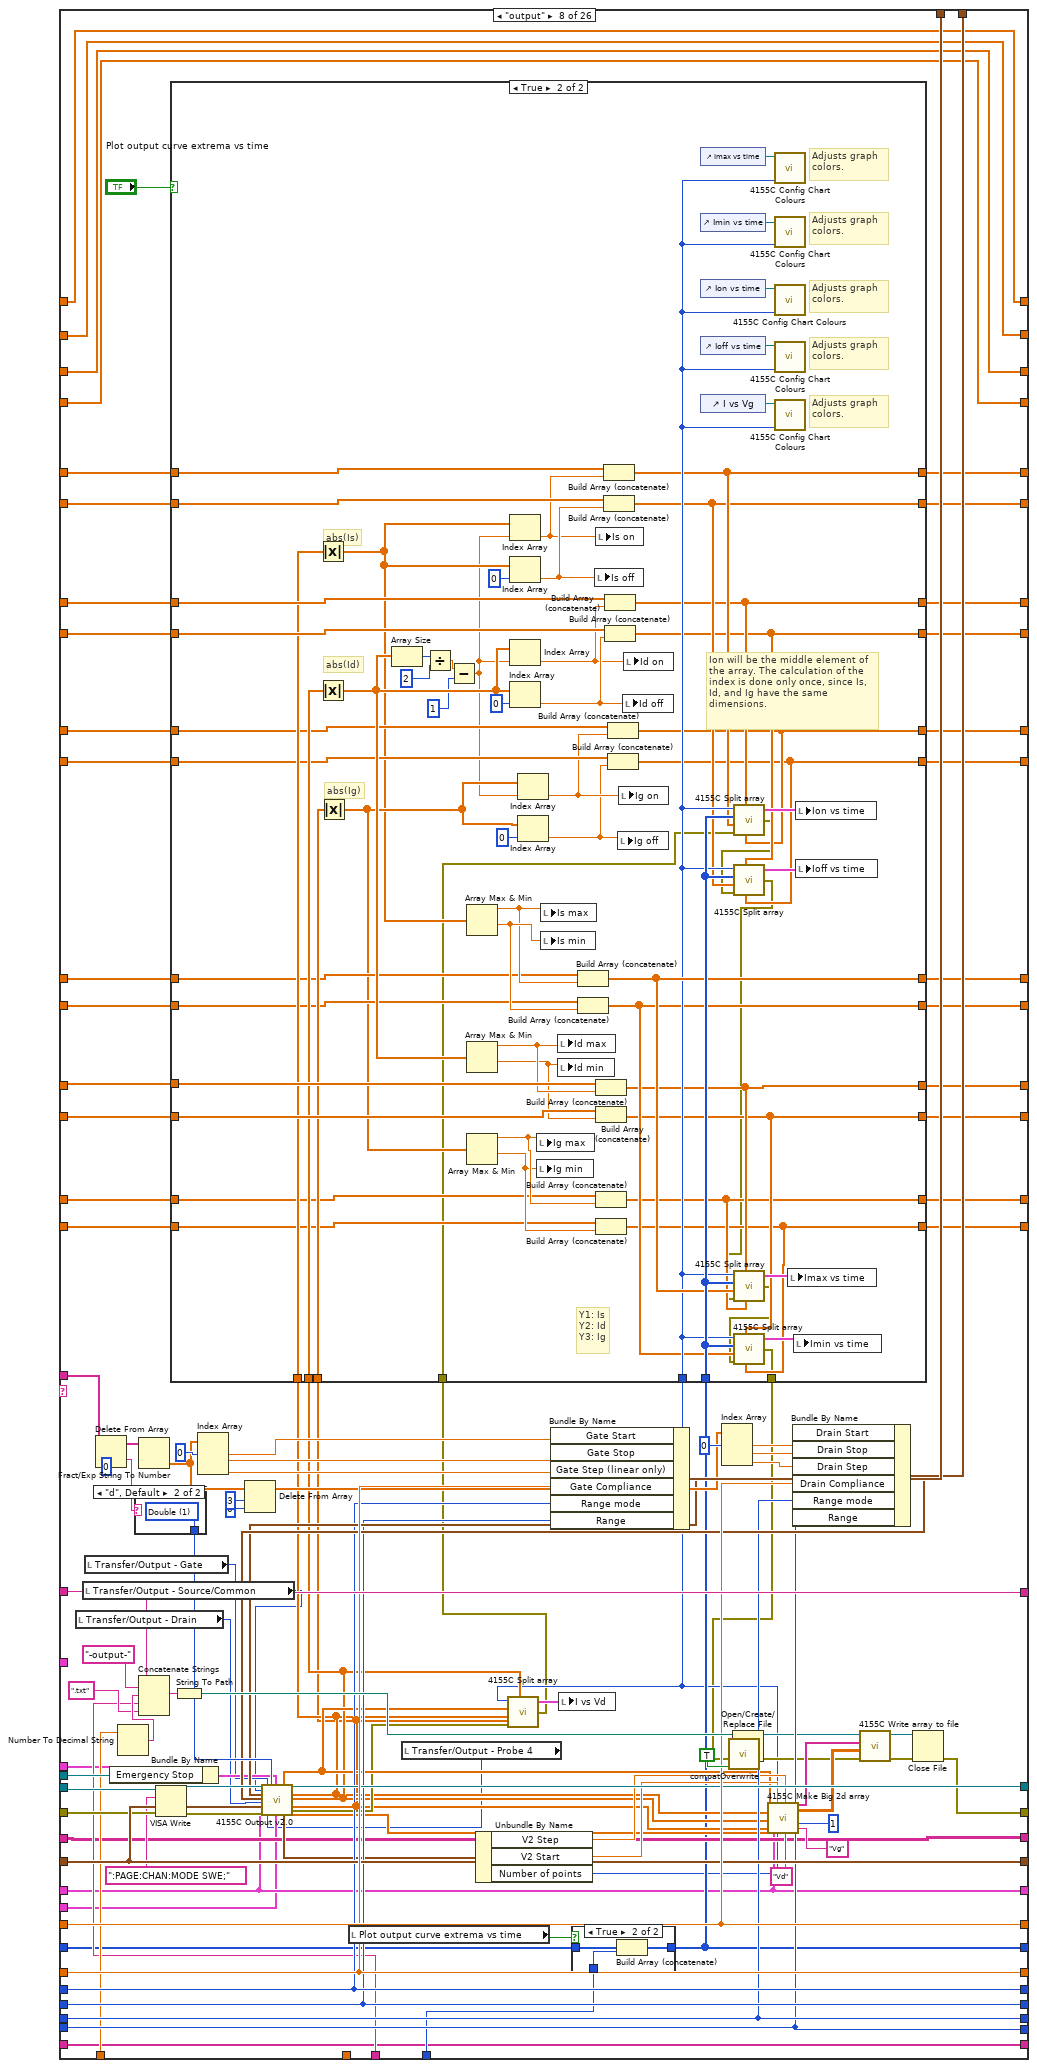
[diagram p19: hidden frame]
diagram:
  w2 = cluster{"Y data in":dbl[], "X data in":dbl[]}[] [] ("I vs Vg")
  w10 = 0.0 ("Is off")
  w11 = 0.0 ("Is on")
  w12 = 0.0 ("Is min")
  w13 = 0.0 ("Is max")
  w58 = u16 1 items=["Reset All", "Partial reset"] ("Type of reset")
  # "Change from previous version:\n\n- Corrected bias stress time axis."
  # "I add 1 to both the \"total lines\" and the \"line running\" indicators because i and N begin from 0, and the script lines begin from 1."
  # "Bugs:\n\n- If using the \"filename\" command, keep in mind that the arrays of the time-dependent data are not re-initialized inbetween filename changes. \n\n- Do not connect the \"error\" wire of a Split block if it has unconnected terminals! It will halt the program."
  # "Array size"
  # "%s option converts a spreadsheet string to an array of strings."
  # "0: No of rows of array\n1: No of cols"
  # "Dimitrios Simatos\nv. 6.9"
  # "Changes from original textcontrol.vi:\n\n- Timestamp appears in filename.\n- (Only) transfer and output curves are plotted.\n- Communication with serial port.\n- Can execute any command, as all pattern matching functions were replaced. Previously, commands with special LabVIEW characters could not be executed.\n- Replaced write to file function with write to text file.\n- Replaced while loop with for loop.\n- Replaced 4155C \"Save File\" function and now the vi can save time-dependent variables.\n- Added clock with start time control and various units.\n- Changed filepath in which the program is saved.\n- Added a serial output log that keeps a history.\n- Tab control.\n- Added option for plotting transfer and output curve extrema vs time.\n- Corrected bug of \"itime\" command. The command did not allow for settting the integration time value, it allowed to set the category of the integration time (short, medium, long). If the time value was beyond the range of the category, then the SPA used the closest value allowed, whilst staying in the category. So, if the integration time was changed to long, but the integration time value was a short one, then the SPA would measure using the minimum long integration time value and not the value that the user intended.\n- Added SMU4 command.\n- Added plotting of \"sample\" plots.\n- Added SMU control."
  # "Search and replace LF with EOL"
  n1 = Equal?(x="integration time", y=u32 0) -> (x = y?=w59:bool)
  n2 = Select(t="Integration time (short)", s=w59, f="Integration time (long)") -> (s? t:f=w18:dbl)
  n3 = call "4155C Get Filename.vi"("error in (no error)"=errorcluster {"status"=FALSE, "code"=0, "source"=""}) -> ("error out"=w53:errorcluster, "path"=w28:path)  [unwired: 2 in, 1 out]
  "Path" <- w28
  n4 = Bundle By Name(cluster="Timings (overwritten by the Front Panel)", "integration time"="integration time", "Short/Long integration time"=w18) -> (w51:T4)
  n5 = Path To String(path=w28) -> (string=w29:string)
  n6 = Match Pattern(string=w29, regular expression=".txt") -> (before substring=w16:string)  [unwired: 1 in, 3 out]
  n7 = Search and Replace String(replace all?=TRUE ("replace all? (F)"), input string="Script", search string="\n", replace string="\r\n") -> (result string=w41:string)  [unwired: 4 in, 3 out]
  n8 = call "4155C Initialise.vi"("VISA resource name in"="VISA resource name in", "Reset"="Full Reset", "Type of reset"=w58, "error in (no error)"=w53, "VISA Timeout Value"=u32 10000) -> ("VISA Resource Name out"=w52:refnum<visa-resource-name>, "error out"=w8:errorcluster)
  n9 = Concatenate Strings(w16, "-script.txt" ("string")) -> (w17:string)
  n10 = String To Path(string=w17) -> (path=w6:path)
  n11 = Spreadsheet String To Array(delimiter (Tab)="\r\n", format string="%s", spreadsheet string="Script", array type (2D Dbl)="") -> (array=w32:string[][])
  n12 = Open/Create/Replace File(file path (use dialog)=w6, error in=w8, operation (0:open)=T8."replace or create with confirmation") -> (refnum out=w5:refnum<file>, error out=w7:errorcluster)  [unwired: 3 in, 1 out]
  n13 = Array Size(array=w32) -> (size(s)=w36:i32[])
  n14 = Initialize Array("") -> (w22:string[])  [unwired: 1 in]
  n15 = Initialize Array("") -> (w20:string[][])  [unwired: 2 in]
  n16 = Initialize Array(0.0 ("element")) -> (w1:dbl[])  [unwired: 1 in]
  n17 = Index Array(array=w36, index=0) -> (element=w34:i32)
  n18 = Write to Text File(file (use dialog)=w5, text=w41, error in=w7) -> (error out=w25:errorcluster)  [unwired: 1 in, 2 out]
  n19 = for {
    N: w34 -> [w160]
    shift-left: "Source/Drain Range" -> [w200]
    shift-right: [w196] -> _
    shift-left: "Source/Drain\nRange mode" -> [w201]
    shift-right: [w197] -> _
    shift-left: "Gate Range" -> [w202]
    shift-right: [w198] -> _
    shift-left: "Gate Range\nmode" -> [w203]
    shift-right: [w199] -> _
    shift-left: "Gate: Compliance" -> [w212]
    shift-right: [w208] -> _
    shift-left: "Drain: Compliance" -> [w213]
    shift-right: [w209] -> _
    shift-left: w51 -> [w214]
    shift-right: [w210] -> w19
    shift-left: w25 -> [w215]
    shift-right: [w70] -> w27
    shift-left: w52 -> [w216]
    shift-right: [w211] -> _
    shift-left: w16 -> [w217]
    shift-right: [w69] -> _
    tunnel: "Panel Controls 2" -> [w194]
    shift-right: [w112] -> _
    shift-left: w1 -> [w193]
    shift-right: [w147] -> _
    shift-left: i32[] [] -> [w189]
    tunnel: w32 -> [w188] mode=indexing
    shift-right: [w111] -> _
    shift-left: w1 -> [w165]
    shift-right: [w142] -> _
    shift-left: w22 -> [w152]
    shift-right: [w143] -> _
    shift-left: w20 -> [w145]
    shift-right: [w105] -> _
    shift-left: w1 -> [w133]
    shift-right: [w106] -> _
    shift-left: w1 -> [w132]
    shift-right: [w110] -> _
    shift-left: w1 -> [w121]
    shift-right: [w109] -> _
    shift-left: w1 -> [w120]
    shift-right: [w103] -> _
    shift-left: w1 -> [w119]
    shift-right: [w113] -> _
    shift-left: w1 -> [w118]
    shift-right: [w104] -> _
    shift-left: w1 -> [w117]
    shift-right: [w102] -> _
    shift-left: w1 -> [w116]
    shift-right: [w108] -> _
    shift-left: w1 -> [w115]
    shift-right: [w107] -> _
    shift-left: w1 -> [w114]
    shift-right: [w95] -> w3
    shift-left: "Probe 4" -> [w195]
    shift-right: [w65] -> _
    shift-left: w1 -> [w92]
    shift-right: [w66] -> _
    shift-left: w1 -> [w91]
    shift-right: [w67] -> _
    shift-left: w1 -> [w90]
    shift-right: [w68] -> _
    shift-left: w1 -> [w89]
    i -> [w155]
    stop <- "Interrupt program" stop-if-true
    # "Ig for bias stress plots"
    # "Id for bias stress plots"
    # "Is for bias stress plots"
    # "Time axis for bias stress plots"
    # "Save bias stress curves in file."
    # "Is off"
    # "Is on"
    # "Ig off"
    # "Ig on"
    # "Is min"
    # "Is max"
    # "Ig min"
    # "Ig max"
    # "Id min"
    # "Id max"
    # "Id off"
    # "Id on"
    # "Is off"
    # "Is on"
    # "Ig off"
    # "Ig on"
    # "Is min"
    # "Is max"
    # "Ig min"
    # "Ig max"
    # "Id min"
    # "Id max"
    # "Id off"
    # "Id on"
    # "Filepath and name"
    # "Limit of command arguments (array columns). Raise if needed."
    # "Serial port data (string)"
    # "Serial port data (table)"
    # "Serial port data"
    # "For loop counter"
    # "<-----Equivalent to the 4155C \"Write\" subvi.----->"
    # "Headers"
    # "Save transfer curves in file."
    # "Filepath and name"
    # "Save time-dependent data."
    # "Use the time offset if your measurements do not start at t=0."
    # "Time for Imax, Imin, Ion, Ioff"
    # "Rest of elements of command"
    # "First element of command\n(case select)"
    n20 = Add(x=w155, y=1) -> (x+y=→"Line running":i32)
    n21 = Add(x=w160, y=1) -> (x+y=→"Total lines":i32)
    n22 = Index Array(array=w188, index=0 ("line index")) -> (element=w183:string)
    "Command running:" <- w183
    n23 = control-ref of="Interrupt scan"() -> (w207:refnum<vi>)
    n24 = Spreadsheet String To Array(delimiter (Tab)=" ", format string="%s", spreadsheet string=w183, array type (2D Dbl)=string[] []) -> (array=w181:string[])
    n25 = Delete From Array(array=w181, index=0) -> (deleted portion=w134:string, array with subset deleted=w180:string[])  [unwired: 1 in]
    n26 = call "Elapsed Time"("Reset"="Reset", "Auto Reset"="Auto Reset") -> ("Elapsed Time (s)"=w190:dbl)  [unwired: 10 in, 7 out]
    n27 = case shown="2" "Time Units" {
      tunnel: ["-sec" "-min" "-h"] -> w191
      tunnel: [w221 w225 w228] -> w161
      tunnel: w190 -> [w221 w224 w229]
      frame 0, Default {
      }
      frame 1 {
        n28 = Divide(x=w224, y=60.0) -> (x/y=w225:dbl)
      }
      frame 2 {
        n29 = Divide(x=w229, y=3600.0) -> (x/y=w228:dbl)
      }
    }
    n30 = Add(x=w161, y="Time Offset") -> (x+y=w93:dbl)
    n31 = To Long Integer(number=w93) -> (32bit integer=w94:i32)
    "Elapsed Time" <- w94
    n32 = case shown="\"sample\"" w134 {
      tunnel: w180 -> [w265 w302 w338 w354 w480 w597 w741 w865 w1030 w1062 w1135 w1180 w1223 w1262 w1294 _ _ w1479 w1617 _ w1721 w1785 w1846 w1939 w2019 w2057]
      tunnel: w217 -> [w260 w298 w336 w367 w487 w656 w749 w872 w1038 w1079 w1124 w1172 w1216 w1256 w1287 w1324 w1384 w1460 w1599 w1648 w1708 w1772 w1834 w1933 w2015 w2059]
      tunnel: w216 -> [w259 w297 w327 w366 w458 w641 w718 w843 w1006 w1080 w1125 w1173 w1217 w1257 w1288 w1329 w1386 w1485 w1623 w1652 w1727 w1791 w1852 w1945 w1973 w2063]
      tunnel: w215 -> [w258 w296 w326 w365 w457 w640 w717 w842 w1003 w1081 w1126 w1174 w1218 w1258 w1289 w1328 w1357 w1484 w1622 w1651 w1726 w1790 w1851 w1944 w1972 w2062]
      tunnel: w214 -> [w257 w295 w335 w363 w483 w617 w745 w868 w1034 w1089 w1134 w1171 w1215 w1255 w1286 w1327 w1381 w1452 w1591 w1657 w1701 w1765 w1827 w1932 w2014 w2064]
      tunnel: w213 -> [w256 w294 w334 w362 w485 w654 w747 w870 w1036 w1088 w1133 w1179 w1222 w1261 w1293 w1326 w1366 w1483 w1621 w1660 w1725 w1789 w1850 w1943 w2023 w2065]
      tunnel: w212 -> [w255 w293 w333 w360 w484 w653 w746 w869 w1035 w1087 w1132 w1178 w1221 w1260 w1292 w1325 w1367 w1461 w1600 w1659 w1709 w1773 w1835 w1934 w2016 w2067]
      tunnel: [w259 w297 w325 w366 w482 w651 w743 w867 w1032 w1080 w1125 w1173 w1217 w1257 w1288 w1329 w1386 w1453 w1573 w1650 w1702 w1766 w1828 w1886 w1975 w2063] -> w211
      tunnel: [w258 w296 w324 w365 w481 w650 w742 w866 w1031 w1081 w1126 w1174 w1218 w1258 w1289 w1328 w1356 w1462 w1574 w1649 w1710 w1774 w1836 w1885 w1974 w2061] -> w146
      tunnel: [w257 w295 w335 w363 w483 w613 w745 w868 w1034 w1082 w1127 w1171 w1215 w1255 w1286 w1327 w1381 w1452 w1591 w1657 w1701 w1765 w1827 w1932 w2014 w2064] -> w210
      tunnel: [w256 w294 w334 w362 w485 w654 w747 w870 w1036 w1088 w1133 w1179 w1222 w1261 w1293 w1326 w1366 w1483 w1621 w1660 w1725 w1789 w1850 w1943 w2023 w2065] -> w209
      tunnel: [w255 w293 w333 w360 w484 w653 w746 w869 w1035 w1087 w1132 w1178 w1221 w1260 w1292 w1325 w1367 w1461 w1600 w1659 w1709 w1773 w1835 w1934 w2016 w2067] -> w208
      tunnel: [w260 w298 w336 w367 w487 w656 w749 w872 w1038 w1079 w1124 w1172 w1216 w1256 w1287 w1324 w1384 w1460 w1599 w1648 w1708 w1772 w1834 w1933 w2015 w2059] -> w69
      tunnel: w207 -> [_ _ _ _ w489 w660 w754 w874 w1042 _ _ _ _ _ _ _ _ w1457 w1596 _ w1707 w1771 w1833 w1905 w1991 _]
      tunnel: "Gate" -> [_ _ _ _ w467 w644 w728 w852 w1017 _ _ _ _ _ _ _ _ _ _ _ _ _ _ _ _ _]
      tunnel: "Drain 2" -> [_ _ _ _ w466 w643 w727 w851 w1016 _ _ _ _ _ _ _ _ _ _ _ _ _ _ _ _ _]
      tunnel: "Panel Controls" -> [_ _ _ _ _ _ w726 w778 w1015 _ _ _ _ _ _ _ _ _ _ _ _ _ _ _ _ _]
      tunnel: w203 -> [w254 w292 w332 w359 w451 w634 w711 w836 w1001 w1086 w1131 _ w1214 w1254 w1285 w1323 w1368 w1448 w1587 w1653 w1697 w1761 w1823 w1928 w2010 w2068]
      tunnel: w202 -> [w253 w291 w331 w358 w450 w633 w710 w835 w1000 w1085 w1130 w1177 _ w1245 w1291 w1322 w1369 w1449 w1588 w1654 w1698 w1762 w1824 w1929 w2011 w2069]
      tunnel: w201 -> [w252 w290 w330 w357 w449 w632 w709 w834 w999 w1084 w1129 w1176 w1220 w1259 _ w1321 w1370 w1450 w1589 w1655 w1699 w1763 w1825 w1930 w2012 w2070]
      tunnel: w200 -> [w251 w289 w329 w356 w448 w631 w708 w833 w1002 w1083 w1128 w1175 w1219 _ w1290 w1320 w1371 w1451 w1590 w1656 w1700 w1764 w1826 w1931 w2013 w2071]
      tunnel: [w254 w292 w332 w359 w451 w634 w711 w836 w1001 w1086 w1131 w1170 w1214 w1254 w1285 w1323 w1368 w1448 w1587 w1653 w1697 w1761 w1823 w1928 w2010 w2068] -> w199
      tunnel: [w253 w291 w331 w358 w450 w633 w710 w835 w1000 w1085 w1130 w1177 w1206 w1245 w1291 w1322 w1369 w1449 w1588 w1654 w1698 w1762 w1824 w1929 w2011 w2069] -> w198
      tunnel: [w252 w290 w330 w357 w449 w632 w709 w834 w999 w1084 w1129 w1176 w1220 w1259 w1284 w1321 w1370 w1450 w1589 w1655 w1699 w1763 w1825 w1930 w2012 w2070] -> w197
      tunnel: [w251 w289 w329 w356 w448 w631 w708 w833 w1002 w1083 w1128 w1175 w1219 w1246 w1290 w1320 w1371 w1451 w1590 w1656 w1700 w1764 w1826 w1931 w2013 w2071] -> w196
      tunnel: w195 -> [w235 w270 w307 _ w389 w586 w680 w774 w970 w1059 w1107 w1154 w1190 w1229 w1268 w1304 w1334 w1435 w1553 w1632 w1668 w1736 w1799 w1865 w1950 w2028]
      tunnel: w194 -> [_ _ _ _ w442 w628 _ _ _ _ _ _ _ _ _ _ _ _ _ _ _ _ _ _ _ _]
      tunnel: [w250 w285 w322 w371 w404 w605 w698 w790 w988 w1078 w1122 w1169 w1205 w1244 w1283 w1319 w1352 w1425 w1557 w1647 w1686 w1754 w1817 w1883 w1968 w2060] -> w112
      tunnel: w193 -> [w250 w285 w322 w371 w439 w605 w698 w825 w988 w1078 w1122 w1169 w1205 w1244 w1283 w1319 w1352 w1431 w1557 w1647 w1686 w1754 w1817 w1883 w1968 w2060]
      tunnel: w93 -> [_ _ _ _ w438 w602 w696 w824 w985 _ _ _ _ _ _ _ w1350 w1440 w1569 _ w1683 w1751 w1814 w1880 w1964 _]
      tunnel: w191 -> [_ _ _ _ w435 w601 w694 w821 w984 _ _ _ _ _ _ _ w1348 w1438 w1568 _ w1682 w1750 w1813 w1879 w1965 _]
      tunnel: w94 -> [_ _ _ _ w431 _ _ w817 _ _ _ _ _ _ _ _ _ _ _ _ _ _ _ _ _ _]
      tunnel: [w249 w284 w321 w361 w408 w604 w697 w794 w987 w1077 w1121 w1168 w1204 w1243 w1282 w1318 w1351 w1410 w1571 w1646 w1685 w1753 w1816 w1882 w1967 w2066] -> w147
      tunnel: w189 -> [w249 w284 w321 w361 w434 w604 w697 w820 w987 w1077 w1121 w1168 w1204 w1243 w1282 w1318 w1351 w1412 w1571 w1646 w1685 w1753 w1816 w1882 w1967 w2066]
      tunnel: [w248 w283 w320 w370 w403 w600 w693 w789 w983 w1076 w1120 w1167 w1203 w1242 w1281 w1317 w1347 w1424 w1556 w1645 w1681 w1749 w1812 w1878 w1963 w2055] -> w111
      tunnel: w165 -> [w248 w283 w320 w370 w430 w600 w693 w816 w983 w1076 w1120 w1167 w1203 w1242 w1281 w1317 w1347 w1430 w1556 w1645 w1681 w1749 w1812 w1878 w1963 w2055]
      tunnel: [w247 w282 w319 w355 w423 w599 w692 w809 w982 w1075 w1119 w1166 w1202 w1241 w1280 w1316 w1346 w1437 w1567 w1644 w1680 w1748 w1811 w1877 w1962 w2054] -> w142
      tunnel: w152 -> [w247 w282 w319 w355 w423 w599 w692 w809 w982 w1075 w1119 w1166 w1202 w1241 w1280 w1316 w1346 w1437 w1567 w1644 w1680 w1748 w1811 w1877 w1962 w2053]
      tunnel: [w246 w281 w318 w364 w422 w598 w691 w808 w981 w1074 w1118 w1165 w1201 w1240 w1279 w1315 w1345 w1436 w1566 w1643 w1679 w1747 w1810 w1876 w1961 w2039] -> w143
      tunnel: w145 -> [w246 w281 w318 w364 w422 w598 w691 w808 w981 w1074 w1118 w1165 w1201 w1240 w1279 w1315 w1345 w1436 w1566 w1643 w1679 w1747 w1810 w1876 w1961 w2039]
      tunnel: [w244 w279 w316 w376 w397 w595 w689 w783 w979 w1072 w1117 w1164 w1199 w1238 w1277 w1313 w1343 w1418 w1565 w1642 w1678 w1746 w1808 w1875 w1960 w2038] -> w105
      tunnel: w133 -> [w244 w279 w316 w376 w421 w595 w689 w807 w979 w1072 w1117 w1164 w1199 w1238 w1277 w1313 w1343 w1418 w1565 w1642 w1678 w1746 w1808 w1875 w1960 w2038]
      tunnel: [w245 w280 w317 w377 w398 w596 w690 w784 w980 w1073 w1116 w1163 w1200 w1239 w1278 w1314 w1344 w1419 w1564 w1641 w1677 w1745 w1809 w1874 w1959 w2037] -> w106
      tunnel: w132 -> [w245 w280 w317 w377 w420 w596 w690 w806 w980 w1073 w1116 w1163 w1200 w1239 w1278 w1314 w1344 w1419 w1564 w1641 w1677 w1745 w1809 w1874 w1959 w2037]
      tunnel: [w237 w272 w309 w369 w402 w592 w687 w788 w977 w1065 w1114 w1161 w1197 w1236 w1275 w1311 w1336 w1423 w1555 w1640 w1670 w1738 w1801 w1867 w1954 w2030] -> w110
      tunnel: w121 -> [w237 w272 w309 w369 w416 w592 w687 w802 w977 w1065 w1114 w1161 w1197 w1236 w1275 w1311 w1336 w1429 w1555 w1640 w1670 w1738 w1801 w1867 w1954 w2030]
      tunnel: [w236 w271 w308 w368 w401 w593 w688 w787 w978 w1064 w1115 w1162 w1198 w1237 w1276 w1312 w1335 w1422 w1554 w1639 w1669 w1737 w1800 w1866 w1953 w2029] -> w109
      tunnel: w120 -> [w236 w271 w308 w368 w415 w593 w688 w801 w978 w1064 w1115 w1162 w1198 w1237 w1276 w1312 w1335 w1428 w1554 w1639 w1669 w1737 w1800 w1866 w1953 w2029]
      tunnel: [w239 w274 w311 w373 w407 w591 w685 w793 w975 w1070 w1112 w1159 w1195 w1234 w1273 w1309 w1338 w1427 w1559 w1634 w1672 w1740 w1803 w1869 w1952 w2034] -> w103
      tunnel: w119 -> [w239 w274 w311 w373 w414 w591 w685 w800 w975 w1070 w1112 w1159 w1195 w1234 w1273 w1309 w1338 w1433 w1559 w1634 w1672 w1740 w1803 w1869 w1952 w2034]
      tunnel: [w238 w273 w310 w372 w405 w594 w686 w791 w976 w1071 w1113 w1160 w1196 w1235 w1274 w1310 w1337 w1426 w1558 w1633 w1671 w1739 w1802 w1868 w1951 w2033] -> w113
      tunnel: w118 -> [w238 w273 w310 w372 w413 w594 w686 w799 w976 w1071 w1113 w1160 w1196 w1235 w1274 w1310 w1337 w1432 w1558 w1633 w1671 w1739 w1802 w1868 w1951 w2033]
      tunnel: [w241 w276 w313 w375 w396 w590 w683 w782 w973 w1068 w1110 w1157 w1193 w1232 w1271 w1307 w1340 w1417 w1561 w1636 w1674 w1742 w1805 w1871 w1956 w2036] -> w104
      tunnel: w117 -> [w241 w276 w313 w375 w412 w590 w683 w798 w973 w1068 w1110 w1157 w1193 w1232 w1271 w1307 w1340 w1417 w1561 w1636 w1674 w1742 w1805 w1871 w1956 w2036]
      tunnel: [w240 w275 w312 w374 w395 w589 w684 w781 w974 w1069 w1111 w1158 w1194 w1233 w1272 w1308 w1339 w1416 w1560 w1635 w1673 w1741 w1804 w1870 w1955 w2035] -> w102
      tunnel: w116 -> [w240 w275 w312 w374 w411 w589 w684 w797 w974 w1069 w1111 w1158 w1194 w1233 w1272 w1308 w1339 w1416 w1560 w1635 w1673 w1741 w1804 w1870 w1955 w2035]
      tunnel: [w243 w278 w315 w379 w400 w588 w681 w786 w971 w1066 w1108 w1155 w1191 w1230 w1269 w1305 w1342 w1421 w1563 w1638 w1676 w1744 w1807 w1873 w1958 w2032] -> w108
      tunnel: w115 -> [w243 w278 w315 w379 w410 w588 w681 w796 w971 w1066 w1108 w1155 w1191 w1230 w1269 w1305 w1342 w1421 w1563 w1638 w1676 w1744 w1807 w1873 w1958 w2032]
      tunnel: [w242 w277 w314 w378 w399 w587 w682 w785 w972 w1067 w1109 w1156 w1192 w1231 w1270 w1306 w1341 w1420 w1562 w1637 w1675 w1743 w1806 w1872 w1957 w2031] -> w107
      tunnel: w114 -> [w242 w277 w314 w378 w409 w587 w682 w795 w972 w1067 w1109 w1156 w1192 w1231 w1270 w1306 w1341 w1420 w1562 w1637 w1675 w1743 w1806 w1872 w1957 w2031]
      tunnel: [w235 w270 w307 w345 w389 w586 w680 w774 w970 w1059 w1107 w1154 w1190 w1229 w1268 w1304 w1334 w1435 w1553 w1632 w1668 w1736 w1799 w1865 w1950 w2028] -> w95
      tunnel: w93 -> [_ _ _ _ _ _ _ _ _ _ _ _ _ _ _ _ _ w1406 _ _ _ _ _ _ _ _]
      tunnel: [w234 w269 w306 w344 w388 w585 w679 w773 w969 w1058 w1106 w1153 w1189 w1228 w1267 w1303 w1333 w1397 w1552 w1631 w1667 w1735 w1798 w1864 w1949 w2027] -> w65
      tunnel: [w233 w268 w305 w343 w387 w584 w678 w772 w968 w1057 w1105 w1152 w1188 w1227 w1266 w1302 w1332 w1394 w1551 w1630 w1666 w1734 w1797 w1863 w1948 w2026] -> w66
      tunnel: [w232 w267 w304 w342 w386 w583 w677 w771 w967 w1056 w1104 w1151 w1187 w1226 w1265 w1301 w1331 w1395 w1550 w1629 w1665 w1733 w1796 w1862 w1947 w2025] -> w67
      tunnel: [w231 w266 w303 w341 w385 w582 w676 w770 w966 w1055 w1103 w1150 w1186 w1225 w1264 w1300 w1330 w1396 w1549 w1628 w1664 w1732 w1795 w1861 w1946 w2024] -> w68
      tunnel: w92 -> [w234 w269 w306 w344 w388 w585 w679 w773 w969 w1058 w1106 w1153 w1189 w1228 w1267 w1303 w1333 w1401 w1552 w1631 w1667 w1735 w1798 w1864 w1949 w2027]
      tunnel: w91 -> [w233 w268 w305 w343 w387 w584 w678 w772 w968 w1057 w1105 w1152 w1188 w1227 w1266 w1302 w1332 w1400 w1551 w1630 w1666 w1734 w1797 w1863 w1948 w2026]
      tunnel: w90 -> [w232 w267 w304 w342 w386 w583 w677 w771 w967 w1056 w1104 w1151 w1187 w1226 w1265 w1301 w1331 w1399 w1550 w1629 w1665 w1733 w1796 w1862 w1947 w2025]
      tunnel: w89 -> [w231 w266 w303 w341 w385 w582 w676 w770 w966 w1055 w1103 w1150 w1186 w1225 w1264 w1300 w1330 w1398 w1549 w1628 w1664 w1732 w1795 w1861 w1946 w2024]
      tunnel: "Standby" -> [_ _ _ _ w384 w581 _ w769 _ _ _ _ _ _ _ _ _ w1392 w1548 _ _ _ _ w1860 _ _]
      frame "wait" {
        n33 = Index Array(array=w265, index=0 ("Index")) -> (element=w263:string)
        n34 = Decimal String To Number(string=w263, default (0L)=u32 0) -> (number=w262:u32)  [unwired: 1 in, 1 out]
        n35 = Wait (ms)(milliseconds to wait=w262) -> ()  [unwired: 1 out]
      }
      frame "wait-min" {
        n36 = Index Array(array=w302, index=0 ("Index")) -> (element=w300:string)
        n37 = Decimal String To Number(string=w300, default (0L)=u32 0) -> (number=w288:u32)  [unwired: 1 in, 1 out]
        n38 = Multiply(x=w288, y=u32 60000) -> (x*y=w287:u32)
        n39 = Wait (ms)(milliseconds to wait=w287) -> ()  [unwired: 1 out]
      }
      frame "standby" {
        n40 = Index Array(array=w338, index=0 ("Index")) -> (element=w328:string)
        n41 = case shown="\"off\", Default" w328 {
          tunnel: [":PAGE:SCON:STAN 0" ":PAGE:SCON:STAN 1"] -> w323
          frame "off", Default {
          }
          frame "on" {
          }
        }
        n42 = VISA Write(VISA resource name=w327, write buffer=w323, error in (no error)=w326) -> (VISA resource name out=w325:refnum<visa-resource-name>, error out=w324:errorcluster)  [unwired: 1 out]
      }
      frame "Probe4" {
        n43 = Delete From Array(array=w354, index=0) -> (deleted portion=w348:string, array with subset deleted=w351:string[])  [unwired: 1 in]
        n44 = Equal?(x=w348, y="ON") -> (x = y?=w346:bool)
        n45 = Delete From Array(array=w351, index=0) -> (deleted portion=w350:string)  [unwired: 1 in, 1 out]
        n46 = Fract/Exp String To Number(string=w350) -> (number=w347:dbl)  [unwired: 3 in, 1 out]
        n47 = Bundle(w346, w347) -> (w345:cluster{bool, dbl})  [unwired: 1 in]
      }
      frame "transfer" {
        n48 = local read "Transfer/Output - Gate"() -> (w383:u32)
        n49 = Delete From Array(array=w480, index=0 ("Index")) -> (deleted portion=w478:string, array with subset deleted=w477:string[])  [unwired: 1 in]
        n50 = Bundle By Name(cluster=w442, "Emergency Stop"=w489) -> (w443:T2)
        n51 = Number To Decimal String(number=w438) -> (decimal integer string=w437:string)  [unwired: 1 in]
        n52 = case shown="\"d\", Default" w478 {
          tunnel: [w574 w575] -> w476
          frame "s" {
            w574 = u16 0 items=["Single", "Double"] ("sweep mode")
          }
          frame "d", Default {
            w575 = u16 1 items=["Single", "Double"] ("sweep mode")
          }
        }
        n53 = Fract/Exp String To Number(string=w477) -> (number=w462:dbl[])  [unwired: 3 in, 1 out]
        n54 = Concatenate Strings(w487, "-transfer-" ("Prefix"), w437, w435, ".txt" ("Suffix (transfer)")) -> (w488:string)
        n55 = VISA Write(VISA resource name=w458, write buffer=":PAGE:CHAN:MODE SWE;" ("write buffer (\"\")"), error in (no error)=w457) -> (VISA resource name out=w455:refnum<visa-resource-name>, error out=w456:errorcluster)  [unwired: 1 out]
        n56 = local read "Plot transfer curve extrema vs time"() -> (w390:bool)
        n57 = String To Path(string=w488) -> (path=w486:path)
        n58 = Index Array(array=w462, index #1=0 ("Index")) -> (element #1=w475:dbl, element #2=w474:dbl, element #3=w473:dbl)  [unwired: 2 in]
        n59 = Delete From Array(array=w462, length=3 ("Length"), index=0 ("Index")) -> (array with subset deleted=w460:dbl[])  [unwired: 1 out]
        n60 = local read "Transfer/Output - Drain"() -> (w380:u32)
        n61 = local read "Transfer/Output - Source/Common"() -> (w382:u32)
        n62 = case shown="True" w390 {
          tunnel: w434 -> [w491 w494]
          tunnel: w431 -> [_ w493]
          tunnel: [w491 w492] -> w408
          frame False {
          }
          frame True {
            n63 = Build Array (concatenate)(w494, w493) -> (w492:i32[])
          }
        }
        n64 = local read "Transfer/Output - Probe 4"() -> (w381:u32)
        n65 = Bundle By Name(cluster=w467, "Gate Start"=w475, "Gate Stop"=w474, "Gate Step (linear only)"=w473, "Gate Compliance"=w484, "Range mode"=w451, "Range"=w450) -> (w452:T6)
        n66 = Index Array(array=w460, index #1=0 ("Index")) -> (element #1=w470:dbl, element #2=w469:dbl, element #3=w468:dbl)  [unwired: 2 in]
        n67 = call <vilib>:"compatOverwrite.vi"("overwrite (F)"=TRUE) -> ("overwrite?"=w441:T8)
        n68 = Bundle By Name(cluster=w466, "Drain Start"=w470, "Drain Stop"=w469, "Drain Step"=w468, "Drain Compliance"=w485, "Range mode"=w449, "Range"=w448) -> (w453:T7)
        n69 = call "4155C Transfer v2.0.vi"("VISA resource name in"=w455, "Source/Common"=w382, 2:"Gate"=w452, 3:"Drain"=w453, 4:"Drain"=w380, "Timings"=w483, "error in (no error)"=w456, 7:"Probe 4"=w389, 8:"Gate"=w383, 9:"Probe 4"=w381, "sweep mode"=w476, "Panel Controls"=w443, "Standby"=w384) -> ("VG"=w440:dbl[], "Outparams"=w447:T9, "VISA Resource Name out"=w482:refnum<visa-resource-name>, "IS"=w418:dbl[], "ID"=w419:dbl[], "IG"=w417:dbl[], "error out"=w432:errorcluster, "Probe 4"=w444:dbl[])  [unwired: 7 in]
        n70 = Unbundle By Name(w447) -> ("V2 Step"=w446:dbl, "V2 Start"=w445:dbl, "Number of points"=w406:i32)
        n71 = call "4155C Split array.vi"("Number of VAR2 steps"=w406, "Y2 data in"=w419, "X data in"=w440, "Y1 data in"=w418, "Y3 data in"=w417, "error in (no error)"=w432) -> ("Array of clusters"=w433:cluster{"Y data in":dbl[], "X data in":dbl[]}[], "error out"=w394:errorcluster)  [unwired: 1 in]
        n72 = case shown="True" "Plot transfer curve extrema vs time" {
          tunnel: w439 -> [w497 w573]
          tunnel: w430 -> [w498 w568]
          tunnel: w421 -> [w504 w564]
          tunnel: w420 -> [w505 w563]
          tunnel: w419 -> [_ w560]
          tunnel: w418 -> [_ w558]
          tunnel: w417 -> [_ w557]
          tunnel: w416 -> [w499 w553]
          tunnel: w415 -> [w501 w552]
          tunnel: w414 -> [w495 w549]
          tunnel: w413 -> [w496 w548]
          tunnel: w412 -> [w503 w545]
          tunnel: w411 -> [w502 w544]
          tunnel: w410 -> [w507 w541]
          tunnel: w409 -> [w506 w540]
          tunnel: w408 -> [_ w533]
          tunnel: [w495 w528] -> w407
          tunnel: w406 -> [_ w527]
          tunnel: [w496 w526] -> w405
          tunnel: [w497 w525] -> w404
          tunnel: [w498 w524] -> w403
          tunnel: [w499 w523] -> w402
          tunnel: [w501 w522] -> w401
          tunnel: [w507 w521] -> w400
          tunnel: [w506 w520] -> w399
          tunnel: [w505 w519] -> w398
          tunnel: [w504 w518] -> w397
          tunnel: [w503 w517] -> w396
          tunnel: [w502 w516] -> w395
          tunnel: w394 -> [w500 w515]
          tunnel: [w500 w511] -> w393
          frame False {
          }
          frame True {
            # "Adjusts graph colors."
            # "Adjusts graph colors."
            # "Ion will be the middle element of the array. The calculation of the index is done only once, since Is, Id, and Ig have the same dimensions."
            # "abs(Ig)"
            # "abs(Is)"
            # "Y1: Is\nY2: Id\nY3: Ig"
            # "abs(Id)"
            # "Adjusts graph colors."
            # "Adjusts graph colors."
            # "Adjusts graph colors."
            n73 = Absolute Value(x=w558) -> (abs(x)=w543:dbl[])
            n74 = Absolute Value(x=w560) -> (abs(x)=w559:dbl[])
            n75 = Absolute Value(x=w557) -> (abs(x)=w546:dbl[])
            n76 = Array Size(array=w559) -> (size(s)=w567:i32)
            n77 = Divide(x=w567, y=2) -> (x/y=w510:dbl)
            n78 = Subtract(x=w510, y=1) -> (x-y=w509:dbl)
            n79 = Array Max & Min(array=w543) -> (max value=w550:dbl, min value=w551:dbl)  [unwired: 2 out]
            n80 = Array Max & Min(array=w559) -> (max value=w572:dbl, min value=w556:dbl)  [unwired: 2 out]
            n81 = Array Max & Min(array=w546) -> (max value=w555:dbl, min value=w554:dbl)  [unwired: 2 out]
            n82 = Index Array(array=w543, index=w509) -> (element=w534:dbl)
            n83 = Index Array(array=w543, index=0) -> (element=w535:dbl)
            n84 = Index Array(array=w559, index=w509) -> (element=w536:dbl)
            n85 = Index Array(array=w559, index=0) -> (element=w537:dbl)
            n86 = Index Array(array=w546, index=w509) -> (element=w539:dbl)
            n87 = Index Array(array=w546, index=0) -> (element=w538:dbl)
            n88 = local write "Ig max"(w555) -> ()
            n89 = local write "Ig min"(w554) -> ()
            n90 = local write "Is max"(w550) -> ()
            n91 = local write "Is min"(w551) -> ()
            n92 = local write "Id max"(w572) -> ()
            n93 = local write "Id min"(w556) -> ()
            n94 = Build Array (concatenate)(w549, w550) -> (w528:dbl[])
            n95 = Build Array (concatenate)(w548, w551) -> (w526:dbl[])
            n96 = local write "Is off"(w535) -> ()
            n97 = local write "Is on"(w534) -> ()
            n98 = Build Array (concatenate)(w573, w572) -> (w525:dbl[])
            n99 = Build Array (concatenate)(w568, w556) -> (w524:dbl[])
            n100 = Build Array (concatenate)(w553, w555) -> (w523:dbl[])
            n101 = Build Array (concatenate)(w552, w554) -> (w522:dbl[])
            n102 = Build Array (concatenate)(w541, w534) -> (w521:dbl[])
            n103 = Build Array (concatenate)(w540, w535) -> (w520:dbl[])
            n104 = Build Array (concatenate)(w563, w536) -> (w519:dbl[])
            n105 = Build Array (concatenate)(w564, w537) -> (w518:dbl[])
            n106 = Build Array (concatenate)(w545, w539) -> (w517:dbl[])
            n107 = Build Array (concatenate)(w544, w538) -> (w516:dbl[])
            n108 = local write "Ig off"(w538) -> ()
            n109 = local write "Ig on"(w539) -> ()
            n110 = local write "Id off"(w537) -> ()
            n111 = local write "Id on"(w536) -> ()
            n112 = control-ref of="Imax vs time"() -> (w562:refnum<vi>)
            n113 = control-ref of="Imin vs time"() -> (w561:refnum<vi>)
            n114 = control-ref of="Ion vs time"() -> (w530:refnum<vi>)
            n115 = control-ref of="Ioff vs time"() -> (w529:refnum<vi>)
            n116 = control-ref of="I vs Vg"() -> (w571:refnum<vi>)
            n117 = call "4155C Split array.vi"("Number of VAR2 steps"=w527, "Y2 data in"=w519, "X data in"=w533, "Y1 data in"=w521, "Y3 data in"=w517, "error in (no error)"=w515) -> ("Array of clusters"=w531:cluster{"Y data in":dbl[], "X data in":dbl[]}[], "error out"=w514:errorcluster)  [unwired: 1 in]
            n118 = call "4155C Split array.vi"("Number of VAR2 steps"=w527, "Y2 data in"=w518, "X data in"=w533, "Y1 data in"=w520, "Y3 data in"=w516, "error in (no error)"=w514) -> ("Array of clusters"=w532:cluster{"Y data in":dbl[], "X data in":dbl[]}[], "error out"=w513:errorcluster)  [unwired: 1 in]
            n119 = call "4155C Split array.vi"("Number of VAR2 steps"=w527, "Y2 data in"=w525, "X data in"=w533, "Y1 data in"=w528, "Y3 data in"=w523, "error in (no error)"=w513) -> ("Array of clusters"=w570:cluster{"Y data in":dbl[], "X data in":dbl[]}[], "error out"=w512:errorcluster)  [unwired: 1 in]
            n120 = call "4155C Split array.vi"("Number of VAR2 steps"=w527, "Y2 data in"=w524, "X data in"=w533, "Y1 data in"=w526, "Y3 data in"=w522, "error in (no error)"=w512) -> ("Array of clusters"=w569:cluster{"Y data in":dbl[], "X data in":dbl[]}[], "error out"=w511:errorcluster)  [unwired: 1 in]
            n121 = call "4155C Config Chart Colours.vi"("Numeric"=w527, "XY Graph 2"=w562) -> ()  [unwired: 6 in]
            n122 = call "4155C Config Chart Colours.vi"("Numeric"=w527, "XY Graph 2"=w561) -> ()  [unwired: 6 in]
            n123 = call "4155C Config Chart Colours.vi"("Numeric"=w527, "XY Graph 2"=w530) -> ()  [unwired: 6 in]
            n124 = call "4155C Config Chart Colours.vi"("Numeric"=w527, "XY Graph 2"=w529) -> ()  [unwired: 6 in]
            n125 = call "4155C Config Chart Colours.vi"("Numeric"=w527, "XY Graph 2"=w571) -> ()  [unwired: 6 in]
            n126 = local write "Imax vs time"(w570) -> ()
            n127 = local write "Imin vs time"(w569) -> ()
            n128 = local write "Ion vs time"(w531) -> ()
            n129 = local write "Ioff vs time"(w532) -> ()
          }
        }
        n130 = local write "I vs Vg"(w433) -> ()
        n131 = Open/Create/Replace File(file path (use dialog)=w486, error in=w393, operation (0:open)=w441) -> (refnum out=w428:refnum<file>, error out=w426:errorcluster)  [unwired: 3 in, 1 out]
        n132 = call "4155C Make Big 2d array.vi"("1D Var1"=w440, "1d IS"=w418, "1d ID"=w419, "1d IG"=w417, "1d SMU4"=w444, "SMU4"=w389, "VAR2 START"=w445, "Number of VAR2 steps"=w406, "VAR2 STEP"=w446, "VAR1 Name"="Vg", "Decimal places in header"=i8 1, "VAR2 Name"="Vd") -> ("Header array"=w429:string[], "Data array"=w427:dbl[][])  [unwired: 14 in]
        n133 = call "4155C Write array to file.vi"("Byte Stream File Refnum"=w428, "Header"=w429, "Data Array"=w427, "error in (no error)"=w426) -> ("dup refnum"=w425:refnum<file>, "error out"=w424:errorcluster)  [unwired: 1 in]
        n134 = Close File(refnum=w425, error in=w424) -> (error out=w481:errorcluster)  [unwired: 1 out]
      }
      frame "pulsedstressV" {
        w611 = 0
        n135 = local read "Pulsed Stress V - Drain"() -> (w580:u32)
        n136 = local read "Pulsed Stress V - Gate"() -> (w577:u32)
        n137 = local read "Pulsed Stress V - Probe 4"() -> (w579:u32)
        n138 = local read "Pulsed Stress V - Source/Common"() -> (w576:u32)
        n139 = local read "Pulsed Stress V - Vextra"() -> (w578:u32)
        n140 = Number To Decimal String(number=w602) -> (decimal integer string=w657:string)  [unwired: 1 in]
        n141 = Delete From Array(array=w597, index=0 ("Index")) -> (deleted portion=w648:string, array with subset deleted=w647:string[])  [unwired: 1 in]
        n142 = Bundle By Name(cluster=w628, "Emergency Stop"=w660) -> (w629:T2)
        n143 = VISA Write(VISA resource name=w641, write buffer=":PAGE:CHAN:MODE SWE;" ("write buffer (\"\")"), error in (no error)=w640) -> (VISA resource name out=w638:refnum<visa-resource-name>, error out=w639:errorcluster)  [unwired: 1 out]
        n144 = Concatenate Strings(w656, "-pulsedstressV-" ("Substring"), w657, w601, ".txt" ("Substring")) -> (w659:string)
        n145 = case shown="\"d\", Default" w648 {
          tunnel: [w669 w670] -> w646
          frame "s" {
            w669 = u16 0 items=["Single", "Double"] ("sweep mode")
          }
          frame "d", Default {
            w670 = u16 1 items=["Single", "Double"] ("sweep mode")
          }
        }
        n146 = Fract/Exp String To Number(string=w647) -> (number=w642:dbl[])  [unwired: 3 in, 1 out]
        n147 = String To Path(string=w659) -> (path=w655:path)
        n148 = Index Array(array=w642, index #1=0 ("Index")) -> (element #1=w620:dbl, element #2=w619:dbl, element #3=w616:dbl, element #4=w615:dbl, element #5=w614:dbl, element #6=w618:dbl)  [unwired: 5 in]
        n149 = Bundle By Name(cluster=w617, "Pulse period"=w615, "Base voltage"=w616, "Pulse width"=w614) -> (w613:T4)
        n150 = Unbundle By Name(w613) -> ("Pulse period"=w621:dbl)
        n151 = Bundle By Name(cluster=w644, "Gate Start"=w619, "Gate Stop"=w620, "Gate Step (linear only)"=0, "Gate Compliance"=w653, "Range mode"=w634, "Range"=w633) -> (w635:T6)
        n152 = call <vilib>:"compatOverwrite.vi"("overwrite (F)"=TRUE) -> ("overwrite?"=w606:T8)
        n153 = Bundle By Name(cluster=w643, "Drain Start"=w618, "Drain Stop"=w611, "Drain Step"=w611, "Drain Compliance"=w654, "Range mode"=w632, "Range"=w631) -> (w636:T7)
        n154 = call "4155C PulsedStressV v2.0.vi"("VISA resource name in"=w638, "Gate"=w635, "Pulsed Stress V - Source/Common"=w576, "Drain"=w636, "Timings"=w613, "error in (no error)"=w639, "sweep mode"=w646, "Probe 4"=w586, "Pulsed Stress V - Drain"=w580, "Pulsed Stress V - Gate"=w577, "Panel Controls"=w629, "Standby"=w581, "Pulsed Stress V - Probe 4"=w579, "Pulsed Stress V - Vextra"=w578) -> ("Outparams"=w630:T9, "VISA Resource Name out"=w651:refnum<visa-resource-name>, "ID"=w609:dbl[], "IG"=w607:dbl[], "error out"=w652:errorcluster)  [unwired: 1 in]
        n155 = Unbundle By Name(w630) -> ("Number of points"=w608:i32)  [unwired: 2 out]
        n156 = for {
          N: w608 -> [_]
          tunnel: [w666] -> w610 mode=indexing
          tunnel: w621 -> [w668]
          i -> [w667]
          n157 = Multiply(x=w668, y=w667) -> (x*y=w666:dbl)
        }
        n158 = Insert Into Array(array=dbl[][] [] ("Input Array"), new element=w610) -> (w622:dbl[][])  [unwired: 2 in]
        n159 = Insert Into Array(array=w622, new element=w609) -> (w627:dbl[][])  [unwired: 2 in]
        n160 = Insert Into Array(array=w627, new element=w607) -> (w626:dbl[][])  [unwired: 2 in]
        n161 = Transpose 2D Array(2D array=w626) -> (transposed array=w625:dbl[][])
        n162 = Open/Create/Replace File(file path (use dialog)=w655, error in=w652, operation (0:open)=w606) -> (refnum out=w663:refnum<file>, error out=w664:errorcluster)  [unwired: 3 in, 1 out]
        n163 = call "4155C Write array to file.vi"("Byte Stream File Refnum"=w663, "Header"=string[] ["Time /s", "Id /A", "Ig /A"], "Data Array"=w625, "error in (no error)"=w664) -> ("dup refnum"=w661:refnum<file>, "error out"=w662:errorcluster)  [unwired: 1 in]
        n164 = Close File(refnum=w661, error in=w662) -> (error out=w650:errorcluster)  [unwired: 1 out]
      }
      frame "transfer-fpp" {
        n165 = local read "FPP - Source"() -> (w675:u32)
        n166 = local read "FPP - Drain"() -> (w673:u32)
        n167 = local read "FPP - Gate"() -> (w674:u32)
        n168 = local read "FPP - Probe 1"() -> (w671:u32)
        n169 = local read "FPP - Probe 2"() -> (w672:u32)
        n170 = Number To Decimal String(number=w696) -> (decimal integer string=w750:string)  [unwired: 1 in]
        n171 = Bundle By Name(cluster=w726, "Emergency Stop"=w754) -> (w762:T1)
        n172 = Delete From Array(array=w741, index=0 ("Index")) -> (deleted portion=w739:string, array with subset deleted=w738:string[])  [unwired: 1 in]
        n173 = Concatenate Strings(w749, "-transferfpp-" ("Substring"), w750, w694, ".txt" ("Substring")) -> (w752:string)
        n174 = VISA Write(VISA resource name=w718, write buffer=":PAGE:CHAN:MODE SWE;" ("write buffer (\"\")"), error in (no error)=w717) -> (VISA resource name out=w715:refnum<visa-resource-name>, error out=w716:errorcluster)  [unwired: 1 out]
        n175 = case shown="\"d\", Default" w739 {
          tunnel: [w763 w764] -> w737
          frame "s" {
            w763 = u16 0 items=["Single", "Double"] ("sweep mode")
          }
          frame "d", Default {
            w764 = u16 1 items=["Single", "Double"] ("sweep mode")
          }
        }
        n176 = Fract/Exp String To Number(string=w738) -> (number=w722:dbl[])  [unwired: 3 in, 1 out]
        n177 = String To Path(string=w752) -> (path=w748:path)
        n178 = Index Array(array=w722, index #1=0 ("Index")) -> (element #1=w736:dbl, element #2=w735:dbl, element #3=w734:dbl)  [unwired: 2 in]
        n179 = Delete From Array(array=w722, length=3 ("Length"), index=0 ("Index")) -> (array with subset deleted=w720:dbl[])  [unwired: 1 out]
        n180 = Bundle By Name(cluster=w728, "Gate Start"=w736, "Gate Stop"=w735, "Gate Step (linear only)"=w734, "Gate Compliance"=w746, "Range mode"=w711, "Range"=w710) -> (w712:T6)
        n181 = Index Array(array=w720, index #1=0 ("Index")) -> (element #1=w731:dbl, element #2=w730:dbl, element #3=w729:dbl)  [unwired: 2 in]
        n182 = call <vilib>:"compatOverwrite.vi"("overwrite (F)"=TRUE) -> ("overwrite?"=w699:T8)
        n183 = Bundle By Name(cluster=w727, "Drain Start"=w731, "Drain Stop"=w730, "Drain Step"=w729, "Drain Compliance"=w747, "Range mode"=w709, "Range"=w708) -> (w713:T7)
        n184 = call "4155C Transfer-FPP v2.0.vi"("VISA resource name in"=w715, "FPP - Source"=w675, "Gate"=w712, "Drain"=w713, "FPP - Drain"=w673, "Timings"=w745, "error in (no error)"=w716, "FPP - Gate"=w674, "FPP - Probe 1"=w671, "sweep mode"=w737, "FPP - Probe 2"=w672, "Panel Controls"=w762) -> ("VG"=w753:dbl[], "Outparams"=w707:T9, "VISA Resource Name out"=w743:refnum<visa-resource-name>, "Vprobe2"=w703:dbl[], "ID"=w702:dbl[], "IG"=w701:dbl[], "Vprobe1"=w700:dbl[], "error out"=w744:errorcluster)  [unwired: 8 in]
        n185 = Unbundle By Name(w707) -> ("V2 Step"=w706:dbl, "V2 Start"=w705:dbl, "Number of points"=w704:i32)
        n186 = Open/Create/Replace File(file path (use dialog)=w748, error in=w744, operation (0:open)=w699) -> (refnum out=w759:refnum<file>, error out=w760:errorcluster)  [unwired: 3 in, 1 out]
        n187 = call "4155C Make Big 2d array FPP.vi"("1D Var1"=w753, "1d ID"=w702, "1d Vp2"=w703, "1d IG"=w701, "1d Vp1"=w700, "VAR2 START"=w705, "Number of VAR2 steps"=w704, "VAR2 STEP"=w706, "VAR1 Name"="Vg", "Decimal places in header"=i8 1, "VAR2 Name"="Vd") -> ("Header array"=w755:string[], "Data array"=w756:dbl[][])  [unwired: 15 in]
        n188 = call "4155C Write array to file.vi"("Byte Stream File Refnum"=w759, "Header"=w755, "Data Array"=w756, "error in (no error)"=w760) -> ("dup refnum"=w757:refnum<file>, "error out"=w758:errorcluster)  [unwired: 1 in]
        n189 = Close File(refnum=w757, error in=w758) -> (error out=w742:errorcluster)  [unwired: 1 out]
      }
      frame "output" {
        n190 = local read "Transfer/Output - Drain"() -> (w766:u32)
        n191 = local read "Transfer/Output - Source/Common"() -> (w765:u32)
        n192 = local read "Transfer/Output - Gate"() -> (w767:u32)
        n193 = Delete From Array(array=w865, index=0 ("Index")) -> (deleted portion=w863:string, array with subset deleted=w862:string[])  [unwired: 1 in]
        n194 = Bundle By Name(cluster=w778, "Emergency Stop"=w874) -> (w828:T1)
        n195 = Number To Decimal String(number=w824) -> (decimal integer string=w823:string)  [unwired: 1 in]
        n196 = case shown="\"d\", Default" w863 {
          tunnel: [w959 w960] -> w861
          frame "s" {
            w959 = u16 0 items=["Single", "Double"] ("sweep mode")
          }
          frame "d", Default {
            w960 = u16 1 items=["Single", "Double"] ("sweep mode")
          }
        }
        n197 = Fract/Exp String To Number(string=w862) -> (number=w847:dbl[])  [unwired: 3 in, 1 out]
        n198 = Concatenate Strings(w872, "-output-" ("Substring"), w823, w821, ".txt" ("Suffix (transfer)")) -> (w873:string)
        n199 = VISA Write(VISA resource name=w843, write buffer=":PAGE:CHAN:MODE SWE;" ("write buffer (\"\")"), error in (no error)=w842) -> (VISA resource name out=w840:refnum<visa-resource-name>, error out=w841:errorcluster)  [unwired: 1 out]
        n200 = String To Path(string=w873) -> (path=w871:path)
        n201 = Index Array(array=w847, index #1=0 ("Index")) -> (element #1=w860:dbl, element #2=w859:dbl, element #3=w858:dbl)  [unwired: 2 in]
        n202 = Delete From Array(array=w847, length=3 ("Length"), index=0 ("Index")) -> (array with subset deleted=w845:dbl[])  [unwired: 1 out]
        n203 = local read "Plot output curve extrema vs time"() -> (w775:bool)
        n204 = local read "Transfer/Output - Probe 4"() -> (w768:u32)
        n205 = Bundle By Name(cluster=w852, "Gate Start"=w860, "Gate Stop"=w859, "Gate Step (linear only)"=w858, "Gate Compliance"=w869, "Range mode"=w836, "Range"=w835) -> (w837:T6)
        n206 = case shown="True" w775 {
          tunnel: w820 -> [w876 w879]
          tunnel: w817 -> [_ w878]
          tunnel: [w876 w877] -> w794
          frame False {
          }
          frame True {
            n207 = Build Array (concatenate)(w879, w878) -> (w877:i32[])
          }
        }
        n208 = Index Array(array=w845, index #1=0 ("Index")) -> (element #1=w855:dbl, element #2=w854:dbl, element #3=w853:dbl)  [unwired: 2 in]
        n209 = call <vilib>:"compatOverwrite.vi"("overwrite (F)"=TRUE) -> ("overwrite?"=w827:T8)
        n210 = Bundle By Name(cluster=w851, "Drain Start"=w855, "Drain Stop"=w854, "Drain Step"=w853, "Drain Compliance"=w870, "Range mode"=w834, "Range"=w833) -> (w838:T7)
        n211 = call "4155C Output v2.0.vi"("VISA resource name in"=w840, "Source/Common"=w765, 2:"Gate"=w837, 3:"Drain"=w838, 4:"Drain"=w766, "Timings"=w868, "error in (no error)"=w841, 7:"Probe 4"=w774, 8:"Gate"=w767, 9:"Probe 4"=w768, "sweep mode"=w861, "Panel controls"=w828, "Standby"=w769) -> ("VD"=w826:dbl[], "Outparams"=w832:T9, "VISA Resource Name out"=w867:refnum<visa-resource-name>, "IS"=w804:dbl[], "ID"=w805:dbl[], "IG"=w803:dbl[], "error out"=w818:errorcluster, "Probe 4"=w829:dbl[])  [unwired: 7 in]
        n212 = Unbundle By Name(w832) -> ("V2 Step"=w831:dbl, "V2 Start"=w830:dbl, "Number of points"=w792:i32)
        n213 = call "4155C Split array.vi"("Number of VAR2 steps"=w792, "Y2 data in"=w805, "X data in"=w826, "Y1 data in"=w804, "Y3 data in"=w803, "error in (no error)"=w818) -> ("Array of clusters"=w819:cluster{"Y data in":dbl[], "X data in":dbl[]}[], "error out"=w780:errorcluster)  [unwired: 1 in]
        n214 = case shown="True" "Plot output curve extrema vs time" {
          tunnel: w825 -> [w888 w958]
          tunnel: w816 -> [w889 w953]
          tunnel: w807 -> [w883 w949]
          tunnel: w806 -> [w882 w948]
          tunnel: w805 -> [_ w945]
          tunnel: w804 -> [_ w943]
          tunnel: w803 -> [_ w942]
          tunnel: w802 -> [w890 w938]
          tunnel: w801 -> [w891 w937]
          tunnel: w800 -> [w886 w934]
          tunnel: w799 -> [w887 w933]
          tunnel: w798 -> [w884 w930]
          tunnel: w797 -> [w885 w929]
          tunnel: w796 -> [w880 w926]
          tunnel: w795 -> [w881 w925]
          tunnel: w794 -> [_ w918]
          tunnel: [w886 w913] -> w793
          tunnel: w792 -> [_ w912]
          tunnel: [w887 w911] -> w791
          tunnel: [w888 w910] -> w790
          tunnel: [w889 w909] -> w789
          tunnel: [w890 w908] -> w788
          tunnel: [w891 w907] -> w787
          tunnel: [w880 w906] -> w786
          tunnel: [w881 w905] -> w785
          tunnel: [w882 w904] -> w784
          tunnel: [w883 w903] -> w783
          tunnel: [w884 w902] -> w782
          tunnel: [w885 w901] -> w781
          tunnel: w780 -> [w892 w900]
          tunnel: [w892 w896] -> w779
          frame False {
          }
          frame True {
            # "Adjusts graph colors."
            # "Adjusts graph colors."
            # "Ion will be the middle element of the array. The calculation of the index is done only once, since Is, Id, and Ig have the same dimensions."
            # "abs(Ig)"
            # "abs(Is)"
            # "Y1: Is\nY2: Id\nY3: Ig"
            # "abs(Id)"
            # "Adjusts graph colors."
            # "Adjusts graph colors."
            # "Adjusts graph colors."
            n215 = Absolute Value(x=w943) -> (abs(x)=w928:dbl[])
            n216 = Absolute Value(x=w945) -> (abs(x)=w944:dbl[])
            n217 = Absolute Value(x=w942) -> (abs(x)=w931:dbl[])
            n218 = Array Size(array=w944) -> (size(s)=w952:i32)
            n219 = Divide(x=w952, y=2) -> (x/y=w895:dbl)
            n220 = Subtract(x=w895, y=1) -> (x-y=w894:dbl)
            n221 = Array Max & Min(array=w928) -> (max value=w935:dbl, min value=w936:dbl)  [unwired: 2 out]
            n222 = Array Max & Min(array=w944) -> (max value=w957:dbl, min value=w941:dbl)  [unwired: 2 out]
            n223 = Array Max & Min(array=w931) -> (max value=w940:dbl, min value=w939:dbl)  [unwired: 2 out]
            n224 = Index Array(array=w928, index=w894) -> (element=w919:dbl)
            n225 = Index Array(array=w928, index=0) -> (element=w920:dbl)
            n226 = Index Array(array=w944, index=w894) -> (element=w921:dbl)
            n227 = Index Array(array=w944, index=0) -> (element=w922:dbl)
            n228 = Index Array(array=w931, index=w894) -> (element=w924:dbl)
            n229 = Index Array(array=w931, index=0) -> (element=w923:dbl)
            n230 = local write "Ig max"(w940) -> ()
            n231 = local write "Ig min"(w939) -> ()
            n232 = local write "Is max"(w935) -> ()
            n233 = local write "Is min"(w936) -> ()
            n234 = local write "Id max"(w957) -> ()
            n235 = local write "Id min"(w941) -> ()
            n236 = Build Array (concatenate)(w934, w935) -> (w913:dbl[])
            n237 = Build Array (concatenate)(w933, w936) -> (w911:dbl[])
            n238 = local write "Is off"(w920) -> ()
            n239 = local write "Is on"(w919) -> ()
            n240 = Build Array (concatenate)(w958, w957) -> (w910:dbl[])
            n241 = Build Array (concatenate)(w953, w941) -> (w909:dbl[])
            n242 = Build Array (concatenate)(w938, w940) -> (w908:dbl[])
            n243 = Build Array (concatenate)(w937, w939) -> (w907:dbl[])
            n244 = Build Array (concatenate)(w926, w919) -> (w906:dbl[])
            n245 = Build Array (concatenate)(w925, w920) -> (w905:dbl[])
            n246 = Build Array (concatenate)(w948, w921) -> (w904:dbl[])
            n247 = Build Array (concatenate)(w949, w922) -> (w903:dbl[])
            n248 = Build Array (concatenate)(w930, w924) -> (w902:dbl[])
            n249 = Build Array (concatenate)(w929, w923) -> (w901:dbl[])
            n250 = local write "Ig off"(w923) -> ()
            n251 = local write "Ig on"(w924) -> ()
            n252 = local write "Id off"(w922) -> ()
            n253 = local write "Id on"(w921) -> ()
            n254 = control-ref of="Imax vs time"() -> (w947:refnum<vi>)
            n255 = control-ref of="Imin vs time"() -> (w946:refnum<vi>)
            n256 = control-ref of="Ion vs time"() -> (w915:refnum<vi>)
            n257 = control-ref of="Ioff vs time"() -> (w914:refnum<vi>)
            n258 = control-ref of="I vs Vg"() -> (w956:refnum<vi>)
            n259 = call "4155C Split array.vi"("Number of VAR2 steps"=w912, "Y2 data in"=w904, "X data in"=w918, "Y1 data in"=w906, "Y3 data in"=w902, "error in (no error)"=w900) -> ("Array of clusters"=w916:cluster{"Y data in":dbl[], "X data in":dbl[]}[], "error out"=w899:errorcluster)  [unwired: 1 in]
            n260 = call "4155C Split array.vi"("Number of VAR2 steps"=w912, "Y2 data in"=w903, "X data in"=w918, "Y1 data in"=w905, "Y3 data in"=w901, "error in (no error)"=w899) -> ("Array of clusters"=w917:cluster{"Y data in":dbl[], "X data in":dbl[]}[], "error out"=w898:errorcluster)  [unwired: 1 in]
            n261 = call "4155C Split array.vi"("Number of VAR2 steps"=w912, "Y2 data in"=w910, "X data in"=w918, "Y1 data in"=w913, "Y3 data in"=w908, "error in (no error)"=w898) -> ("Array of clusters"=w955:cluster{"Y data in":dbl[], "X data in":dbl[]}[], "error out"=w897:errorcluster)  [unwired: 1 in]
            n262 = call "4155C Split array.vi"("Number of VAR2 steps"=w912, "Y2 data in"=w909, "X data in"=w918, "Y1 data in"=w911, "Y3 data in"=w907, "error in (no error)"=w897) -> ("Array of clusters"=w954:cluster{"Y data in":dbl[], "X data in":dbl[]}[], "error out"=w896:errorcluster)  [unwired: 1 in]
            n263 = call "4155C Config Chart Colours.vi"("Numeric"=w912, "XY Graph 2"=w947) -> ()  [unwired: 6 in]
            n264 = call "4155C Config Chart Colours.vi"("Numeric"=w912, "XY Graph 2"=w946) -> ()  [unwired: 6 in]
            n265 = call "4155C Config Chart Colours.vi"("Numeric"=w912, "XY Graph 2"=w915) -> ()  [unwired: 6 in]
            n266 = call "4155C Config Chart Colours.vi"("Numeric"=w912, "XY Graph 2"=w914) -> ()  [unwired: 6 in]
            n267 = call "4155C Config Chart Colours.vi"("Numeric"=w912, "XY Graph 2"=w956) -> ()  [unwired: 6 in]
            n268 = local write "Imax vs time"(w955) -> ()
            n269 = local write "Imin vs time"(w954) -> ()
            n270 = local write "Ion vs time"(w916) -> ()
            n271 = local write "Ioff vs time"(w917) -> ()
          }
        }
        n272 = local write "I vs Vd"(w819) -> ()
        n273 = Open/Create/Replace File(file path (use dialog)=w871, error in=w779, operation (0:open)=w827) -> (refnum out=w814:refnum<file>, error out=w812:errorcluster)  [unwired: 3 in, 1 out]
        n274 = call "4155C Make Big 2d array.vi"("1D Var1"=w826, "1d IS"=w804, "1d ID"=w805, "1d IG"=w803, "1d SMU4"=w829, "SMU4"=w774, "VAR2 START"=w830, "Number of VAR2 steps"=w792, "VAR2 STEP"=w831, "VAR1 Name"="Vd", "Decimal places in header"=i8 1, "VAR2 Name"="Vg") -> ("Header array"=w815:string[], "Data array"=w813:dbl[][])  [unwired: 14 in]
        n275 = call "4155C Write array to file.vi"("Byte Stream File Refnum"=w814, "Header"=w815, "Data Array"=w813, "error in (no error)"=w812) -> ("dup refnum"=w811:refnum<file>, "error out"=w810:errorcluster)  [unwired: 1 in]
        n276 = Close File(refnum=w811, error in=w810) -> (error out=w866:errorcluster)  [unwired: 1 out]
      }
      frame "output-fpp" {
        n277 = local read "FPP - Source"() -> (w963:u32)
        n278 = local read "FPP - Drain"() -> (w964:u32)
        n279 = local read "FPP - Gate"() -> (w965:u32)
        n280 = Number To Decimal String(number=w985) -> (decimal integer string=w1039:string)  [unwired: 1 in]
        n281 = Bundle By Name(cluster=w1015, "Emergency Stop"=w1042) -> (w1052:T1)
        n282 = Delete From Array(array=w1030, index=0 ("Index")) -> (deleted portion=w1028:string, array with subset deleted=w1027:string[])  [unwired: 1 in]
        n283 = VISA Write(VISA resource name=w1006, write buffer=":PAGE:CHAN:MODE SWE;" ("write buffer (\"\")"), error in (no error)=w1003) -> (VISA resource name out=w1005:refnum<visa-resource-name>, error out=w1004:errorcluster)  [unwired: 1 out]
        n284 = Concatenate Strings(w1038, "-outputfpp-" ("Substring"), w1039, w984, ".txt" ("Substring")) -> (w1041:string)
        n285 = case shown="\"d\", Default" w1028 {
          tunnel: [w1053 w1054] -> w1026
          frame "s" {
            w1053 = u16 0 items=["Single", "Double"] ("sweep mode")
          }
          frame "d", Default {
            w1054 = u16 1 items=["Single", "Double"] ("sweep mode")
          }
        }
        n286 = Fract/Exp String To Number(string=w1027) -> (number=w1009:dbl[])  [unwired: 3 in, 1 out]
        n287 = String To Path(string=w1041) -> (path=w1037:path)
        n288 = Index Array(array=w1009, index #1=0 ("Index")) -> (element #1=w1025:dbl, element #2=w1024:dbl, element #3=w1023:dbl)  [unwired: 2 in]
        n289 = Delete From Array(array=w1009, length=3 ("Length"), index=0 ("Index")) -> (array with subset deleted=w1008:dbl[])  [unwired: 1 out]
        n290 = local read "FPP - Probe 1"() -> (w961:u32)
        n291 = local read "FPP - Probe 2"() -> (w962:u32)
        n292 = Bundle By Name(cluster=w1017, "Gate Start"=w1025, "Gate Stop"=w1024, "Gate Step (linear only)"=w1023, "Gate Compliance"=w1035, "Range mode"=w1001, "Range"=w1000) -> (w1051:T6)
        n293 = Index Array(array=w1008, index #1=0 ("Index")) -> (element #1=w1020:dbl, element #2=w1019:dbl, element #3=w1018:dbl)  [unwired: 2 in]
        n294 = call <vilib>:"compatOverwrite.vi"("overwrite (F)"=TRUE) -> ("overwrite?"=w989:T8)
        n295 = Bundle By Name(cluster=w1016, "Drain Start"=w1020, "Drain Stop"=w1019, "Drain Step"=w1018, "Drain Compliance"=w1036, "Range mode"=w999, "Range"=w1002) -> (w1050:T7)
        n296 = call "4155C Output-FPP v2.0.vi"("VISA resource name in"=w1005, "FPP - Source"=w963, "Gate"=w1051, "Drain"=w1050, "FPP - Drain"=w964, "Timings"=w1034, "error in (no error)"=w1004, "FPP - Gate"=w965, "FPP - Probe 1"=w961, "sweep mode"=w1026, "FPP - Probe 2"=w962, "Panel controls"=w1052) -> ("VD"=w994:dbl[], "Outparams"=w997:T9, "VISA Resource Name out"=w1032:refnum<visa-resource-name>, "Vprobe2"=w993:dbl[], "ID"=w992:dbl[], "IG"=w991:dbl[], "Vprobe1"=w990:dbl[], "error out"=w1033:errorcluster)  [unwired: 8 in]
        n297 = Unbundle By Name(w997) -> ("V2 Step"=w998:dbl, "V2 Start"=w996:dbl, "Number of points"=w995:i32)
        n298 = Open/Create/Replace File(file path (use dialog)=w1037, error in=w1033, operation (0:open)=w989) -> (refnum out=w1047:refnum<file>, error out=w1048:errorcluster)  [unwired: 3 in, 1 out]
        n299 = call "4155C Make Big 2d array FPP.vi"("1D Var1"=w994, "1d ID"=w992, "1d Vp2"=w993, "1d IG"=w991, "1d Vp1"=w990, "VAR2 START"=w996, "Number of VAR2 steps"=w995, "VAR2 STEP"=w998, "VAR1 Name"="Vd", "Decimal places in header"=i8 1, "VAR2 Name"="Vg") -> ("Header array"=w1043:string[], "Data array"=w1044:dbl[][])  [unwired: 15 in]
        n300 = call "4155C Write array to file.vi"("Byte Stream File Refnum"=w1047, "Header"=w1043, "Data Array"=w1044, "error in (no error)"=w1048) -> ("dup refnum"=w1045:refnum<file>, "error out"=w1046:errorcluster)  [unwired: 1 in]
        n301 = Close File(refnum=w1045, error in=w1046) -> (error out=w1031:errorcluster)  [unwired: 1 out]
      }
      frame "itime" {
        n302 = Delete From Array(array=w1062, index=1) -> (deleted portion=w1061:string)  [unwired: 1 in, 1 out]
        n303 = Delete From Array(array=w1062, index=0 ("Index")) -> (deleted portion=w1090:string)  [unwired: 1 in, 1 out]
        n304 = Fract/Exp String To Number(string=w1061) -> (number=w1060:dbl)  [unwired: 3 in, 1 out]
        n305 = case shown="\"l\"" w1090 {
          tunnel: w1089 -> [w1095 w1097 w1101]
          tunnel: [w1094 w1096 w1100] -> w1082
          tunnel: w1060 -> [w1092 _ w1099]
          frame "s" {
            w1093 = u32 0 items=["short  ", "medium  ", "long  "] ("integration time 2")
            n306 = Bundle By Name(cluster=w1095, "integration time"=w1093, "Short/Long integration time"=w1092) -> (w1094:T4)
          }
          frame "m", Default {
            w1098 = u32 1 items=["short  ", "medium  ", "long  "] ("integration time 2")
            n307 = Bundle By Name(cluster=w1097, "integration time"=w1098) -> (w1096:T4)
          }
          frame "l" {
            w1102 = u32 2 items=["short  ", "medium  ", "long  "] ("integration time 2")
            n308 = Bundle By Name(cluster=w1101, "integration time"=w1102, "Short/Long integration time"=w1099) -> (w1100:T4)
          }
        }
      }
      frame "pulsed" {
        n309 = Delete From Array(array=w1135, index=0 ("Index")) -> (deleted portion=w1136:string, array with subset deleted=w1123:string[])  [unwired: 1 in]
        n310 = case shown="\"on\", Default" w1136 {
          tunnel: w1134 -> [w1146 w1149]
          tunnel: [w1145 w1148] -> w1127
          tunnel: w1123 -> [w1143 _]
          frame "on", Default {
            w1144 = u16 1 items=["Continuous", "Pulsed"] ("sweep method")
            n311 = Fract/Exp String To Number(string=w1143) -> (number=w1141:dbl[])  [unwired: 3 in, 1 out]
            n312 = Index Array(array=w1141, index #1=0 ("Index")) -> (element #1=w1140:dbl, element #2=w1139:dbl, element #3=w1138:dbl)  [unwired: 2 in]
            n313 = Bundle By Name(cluster=w1146, "sweep method"=w1144, "Pulse period"=w1140, "Base voltage"=w1139, "Pulse width"=w1138) -> (w1145:T4)
          }
          frame "off" {
            w1147 = u16 0 items=["Continuous", "Pulsed"] ("sweep method")
            n314 = Bundle By Name(cluster=w1149, "sweep method"=w1147) -> (w1148:T4)
          }
        }
      }
      frame "gaterangemode" {
        n315 = Delete From Array(array=w1180, index=0 ("Index")) -> (deleted portion=w1181:string)  [unwired: 1 in, 1 out]
        n316 = case shown="\"f\"" w1181 {
          tunnel: [w1183 w1184 w1185] -> w1170
          frame "a", Default {
            w1183 = u16 0 items=["Auto", "Limited", "Fixed"] ("Gate Range\nmode 2")
          }
          frame "f" {
            w1184 = u16 2 items=["Auto", "Limited", "Fixed"] ("Gate Range\nmode 2")
          }
          frame "l" {
            w1185 = u16 1 items=["Auto", "Limited", "Fixed"] ("Gate Range\nmode 2")
          }
        }
      }
      frame "gaterange" {
        (unwired) u8 11 items=["10fA  ", "100fA  ", "1nA  ", "10nA", "100nA", "1uA", "10uA", "100uA", "1mA", "10mA", "100mA", "1A"] ("Gate Range 2")
        n317 = Delete From Array(array=w1223, index=0 ("Index")) -> (deleted portion=w1213:string)  [unwired: 1 in, 1 out]
        n318 = Scan Value(string=w1213, format string="") -> (value=w1211:dbl)  [unwired: 1 in, 1 out]
        n319 = Logarithm Base 10(1:w1211) -> (0:w1210:dbl)
        n320 = Round To Nearest(number=w1210) -> (nearest integer value=w1209:dbl)
        n321 = Add(x=w1209, y=11.0) -> (x+y=w1207:dbl)
        n322 = To Unsigned Byte Integer(number=w1207) -> (unsigned 8bit integer=w1206:u8)
      }
      frame "drainrange" {
        (unwired) u8 11 items=["10fA  ", "100fA  ", "1nA  ", "10nA", "100nA", "1uA", "10uA", "100uA", "1mA", "10mA", "100mA", "1A"] ("Gate Range 2")
        n323 = Delete From Array(array=w1262, index=0 ("Index")) -> (deleted portion=w1253:string)  [unwired: 1 in, 1 out]
        n324 = Scan Value(string=w1253, format string="") -> (value=w1251:dbl)  [unwired: 1 in, 1 out]
        n325 = Logarithm Base 10(1:w1251) -> (0:w1250:dbl)
        n326 = Round To Nearest(number=w1250) -> (nearest integer value=w1249:dbl)
        n327 = Add(x=w1249, y=11.0) -> (x+y=w1247:dbl)
        n328 = To Unsigned Byte Integer(number=w1247) -> (unsigned 8bit integer=w1246:u8)
      }
      frame "drainrangemode" {
        n329 = Delete From Array(array=w1294, index=0 ("Index")) -> (deleted portion=w1295:string)  [unwired: 1 in, 1 out]
        n330 = case shown="\"f\"" w1295 {
          tunnel: [w1297 w1298 w1299] -> w1284
          frame "a", Default {
            w1297 = u16 0 items=["Auto", "Limited", "Fixed"] ("Gate Range\nmode 2")
          }
          frame "f" {
            w1298 = u16 2 items=["Auto", "Limited", "Fixed"] ("Gate Range\nmode 2")
          }
          frame "l" {
            w1299 = u16 1 items=["Auto", "Limited", "Fixed"] ("Gate Range\nmode 2")
          }
        }
      }
      frame "Error", Default {
      }
      frame "logfile" {
        n331 = Number To Decimal String(number=w1350) -> (decimal integer string=w1385:string)  [unwired: 1 in]
        n332 = Concatenate Strings(w1384, "logfile" ("Substring"), w1385, w1348, ".txt" ("Substring")) -> (w1382:string)
        n333 = String To Path(string=w1382) -> (path=w1355:path)
        n334 = Unbundle(w1381) -> ("integration time"=w1380:u32, "Short/Long integration time"=w1379:dbl, "hold time (sec)"=w1378:dbl, "delay time (sec)"=w1377:dbl, "Step Time (0 disables)"=w1376:dbl, "sweep method"=w1375:u16, "Pulse period"=w1374:dbl, "Base voltage"=w1373:dbl, "Pulse width"=w1372:dbl)
        n335 = Build Array(w1380, w1379, w1378, w1377, w1376, w1375, w1374, w1373, w1372, w1366, w1367, w1368, w1369, w1370, w1371) -> (w1359:dbl[])
        n336 = Insert Into Array(array=dbl[][] [] ("Input Array"), new element=w1359) -> (w1358:dbl[][])  [unwired: 2 in]
        n337 = call <vilib>:"compatOverwrite.vi"("overwrite (F)"=TRUE) -> ("overwrite?"=w1353:T8)
        n338 = Open/Create/Replace File(file path (use dialog)=w1355, error in=w1357, operation (0:open)=w1353) -> (refnum out=w1363:refnum<file>, error out=w1362:errorcluster)  [unwired: 3 in, 1 out]
        n339 = call "4155C Write array to file.vi"("Byte Stream File Refnum"=w1363, "Header"=string[] ["Int Time", "Short/Long Itime", "Hold time", "Delay time", "Step time", "Sweep method", "Pulse period", "Base Voltage", "Pulse width", "Drain compliance", "Gate compliance", "Gate range mode", "Gate range", "S/D range mode", "S/D range"], "Data Array"=w1358, "error in (no error)"=w1362) -> ("dup refnum"=w1365:refnum<file>, "error out"=w1364:errorcluster)  [unwired: 1 in]
        n340 = Close File(refnum=w1365, error in=w1364) -> (error out=w1356:errorcluster)  [unwired: 1 out]
      }
      frame "sample" {
        w1408 = 1
        # "Add a time offset (elapsed time) to the time axis."
        # "Adjusts graph colors."
        n341 = Number To Decimal String(number=w1440) -> (decimal integer string=w1482:string)  [unwired: 1 in]
        n342 = Fract/Exp String To Number(string=w1479) -> (number=w1444:dbl[])  [unwired: 3 in, 1 out]
        n343 = local read "Sample - Probe 4"() -> (w1388:u32)
        n344 = Concatenate Strings(w1460, "-sample-" ("Substring"), w1482, w1438, ".txt" ("Substring")) -> (w1480:string)
        n345 = local read "Sample - Drain"() -> (w1389:u32)
        n346 = Index Array(array=w1444, index=0 ("Index")) -> (element=w1477:dbl)
        n347 = String To Path(string=w1480) -> (path=w1464:path)
        n348 = Index Array(array=w1444, index=2 ("Index")) -> (element=w1473:dbl)
        n349 = Index Array(array=w1444, index=3 ("Index")) -> (element=w1446:dbl)
        n350 = Index Array(array=w1444, index=4 ("Index")) -> (element=w1443:dbl)
        n351 = Index Array(array=w1444, index=1 ("Index")) -> (element=w1474:dbl)
        n352 = local read "Plot sample extrema vs time"() -> (w1411:bool)
        n353 = local read "Time Units"() -> (w1387:u16)
        n354 = local read "Sample - Gate"() -> (w1391:u32)
        n355 = local read "Sample - Source/Common"() -> (w1390:u32)
        n356 = call "4155C Config Sampling Measurements v2.0.vi"("VISA session"=w1485, "Num Points"=w1473, "Sample - Drain"=w1389, "Display on/off"=TRUE, "Gate Compliance"=w1461, "Sampling interval"=w1443, "Sample - Source/Common"=w1390, "Sample - Probe 4"=w1388, "Drain Compliance"=w1483, "Standby"=w1392, "error in (no error)"=w1484, "Timings"=w1452, "Sample - Gate"=w1391, "Sample time"=w1446) -> ("dup VISA resource name"=w1487:refnum<visa-resource-name>, "error out"=w1486:errorcluster)
        n357 = call "4155C Take Sample v2.0.vi"("VISA resource name in"=w1487, "Emergency Stop"=w1457, "Sample - Gate"=w1391, "Vg"=w1477, "Sample - Drain"=w1389, "Vd"=w1474, "error in (no error)"=w1486) -> ("Time"=w1407:dbl[], "VISA Resource Name out"=w1454:refnum<visa-resource-name>, "Ig"=w1402:dbl[], "Id"=w1403:dbl[], "Is"=w1404:dbl[], "error out"=w1409:errorcluster)  [unwired: 3 in]
        n358 = case shown="2" w1387 {
          tunnel: w1407 -> [w1492 w1497 w1500]
          tunnel: w1406 -> [w1488 w1493 w1499]
          tunnel: [w1491 w1496 w1498] -> w1405
          frame 1 {
            n359 = Multiply(x=w1488, y=60.0) -> (x*y=w1490:dbl)
            n360 = Add(x=w1492, y=w1490) -> (x+y=w1491:dbl[])
          }
          frame 2 {
            n361 = Multiply(x=w1493, y=3600.0) -> (x*y=w1495:dbl)
            n362 = Add(x=w1497, y=w1495) -> (x+y=w1496:dbl[])
          }
          frame 0, Default {
            n363 = Add(x=w1500, y=w1499) -> (x+y=w1498:dbl[])
          }
        }
        n364 = Insert Into Array(array=w1400, new element=w1403) -> (w1394:dbl[])  [unwired: 1 in]
        n365 = Insert Into Array(array=w1399, new element=w1404) -> (w1395:dbl[])  [unwired: 1 in]
        n366 = Insert Into Array(array=w1401, new element=w1402) -> (w1397:dbl[])  [unwired: 1 in]
        n367 = case shown="True" w1411 {
          tunnel: w1412 -> [w1501 w1503]
          tunnel: [w1501 w1504] -> w1410
          tunnel: w1405 -> [_ w1502]
          frame False {
          }
          frame True {
            n368 = Insert Into Array(array=w1503, new element=w1502) -> (w1504:i32[])  [unwired: 1 in]
          }
        }
        n369 = case shown="True" "Plot sample extrema vs time" {
          tunnel: w1404 -> [_ w1532]
          tunnel: w1403 -> [_ w1533]
          tunnel: w1402 -> [_ w1534]
          tunnel: [w1511 w1521] -> w1393
          tunnel: w1409 -> [w1511 w1525]
          tunnel: w1433 -> [w1510 w1537]
          tunnel: w1432 -> [w1509 w1536]
          tunnel: w1431 -> [w1508 w1538]
          tunnel: w1430 -> [w1507 w1535]
          tunnel: w1429 -> [w1506 w1540]
          tunnel: w1428 -> [w1505 w1539]
          tunnel: [w1510 w1523] -> w1427
          tunnel: [w1509 w1516] -> w1426
          tunnel: [w1508 w1517] -> w1425
          tunnel: [w1507 w1541] -> w1424
          tunnel: [w1506 w1524] -> w1423
          tunnel: [w1505 w1518] -> w1422
          tunnel: w1410 -> [_ w1512]
          frame False {
          }
          frame True {
            w1519 = 1
            # "Number of VAR2 steps is 1."
            # "abs(Ig)"
            # "abs(Is)"
            # "abs(Id)"
            # "Adjusts graph colors."
            n370 = Absolute Value(x=w1534) -> (abs(x)=w1513:dbl[])
            n371 = Absolute Value(x=w1533) -> (abs(x)=w1514:dbl[])
            n372 = Absolute Value(x=w1532) -> (abs(x)=w1515:dbl[])
            n373 = Array Max & Min(array=w1515) -> (max value=w1531:dbl, min value=w1528:dbl)  [unwired: 2 out]
            n374 = Array Max & Min(array=w1514) -> (max value=w1530:dbl, min value=w1527:dbl)  [unwired: 2 out]
            n375 = Array Max & Min(array=w1513) -> (max value=w1529:dbl, min value=w1526:dbl)  [unwired: 2 out]
            n376 = local write "Id max"(w1530) -> ()
            n377 = local write "Id min"(w1527) -> ()
            n378 = local write "Ig max"(w1529) -> ()
            n379 = local write "Ig min"(w1526) -> ()
            n380 = Insert Into Array(array=w1540, new element=w1513) -> (w1524:dbl[])  [unwired: 1 in]
            n381 = Insert Into Array(array=w1539, new element=w1513) -> (w1518:dbl[])  [unwired: 1 in]
            n382 = local write "Is max"(w1531) -> ()
            n383 = local write "Is min"(w1528) -> ()
            n384 = Insert Into Array(array=w1538, new element=w1514) -> (w1517:dbl[])  [unwired: 1 in]
            n385 = Insert Into Array(array=w1535, new element=w1514) -> (w1541:dbl[])  [unwired: 1 in]
            n386 = Insert Into Array(array=w1537, new element=w1515) -> (w1523:dbl[])  [unwired: 1 in]
            n387 = Insert Into Array(array=w1536, new element=w1515) -> (w1516:dbl[])  [unwired: 1 in]
            n388 = control-ref of="Imax vs time"() -> (w1542:refnum<vi>)
            n389 = call "4155C Config Chart Colours.vi"("Numeric"=w1519, "XY Graph 2"=w1542) -> ()  [unwired: 6 in]
            n390 = call "4155C Split array.vi"("Number of VAR2 steps"=w1519, "Y2 data in"=w1517, "X data in"=w1512, "Y1 data in"=w1523, "Y3 data in"=w1524, "error in (no error)"=w1525) -> ("Array of clusters"=w1543:cluster{"Y data in":dbl[], "X data in":dbl[]}[], "error out"=w1522:errorcluster)  [unwired: 1 in]
            n391 = call "4155C Split array.vi"("Number of VAR2 steps"=w1519, "Y2 data in"=w1517, "X data in"=w1512, "Y1 data in"=w1516, "Y3 data in"=w1518, "error in (no error)"=w1522) -> ("Array of clusters"=w1520:cluster{"Y data in":dbl[], "X data in":dbl[]}[], "error out"=w1521:errorcluster)  [unwired: 1 in]
            n392 = local write "Imax vs time"(w1543) -> ()
            n393 = local write "Imin vs time"(w1520) -> ()
          }
        }
        n394 = Insert Into Array(array=w1398, new element=w1405) -> (w1396:dbl[])  [unwired: 1 in]
        n395 = control-ref of="I vs time (Bias Stress)"() -> (w1415:refnum<vi>)
        n396 = call "4155C Split array.vi"("Number of VAR2 steps"=w1408, "Y2 data in"=w1394, "X data in"=w1396, "Y1 data in"=w1395, "Y3 data in"=w1397) -> ("Array of clusters"=w1414:cluster{"Y data in":dbl[], "X data in":dbl[]}[])  [unwired: 2 in, 1 out]
        n397 = call "4155C Config Chart Colours.vi"("Numeric"=w1408, "XY Graph 2"=w1415) -> ()  [unwired: 6 in]
        n398 = local write "I vs time (Bias Stress)"(w1414) -> ()
        n399 = Insert Into Array(array=dbl[][] [] ("Input Array"), new element=w1405) -> (w1413:dbl[][])  [unwired: 2 in]
        n400 = Insert Into Array(array=w1413, new element=w1402) -> (w1467:dbl[][])  [unwired: 2 in]
        n401 = VISA Write(VISA resource name=w1454, write buffer=":DISP ON" ("write buffer (\"\")"), error in (no error)=w1393) -> (VISA resource name out=w1453:refnum<visa-resource-name>, error out=w1455:errorcluster)  [unwired: 1 out]
        n402 = Insert Into Array(array=w1467, new element=w1403) -> (w1466:dbl[][])  [unwired: 2 in]
        n403 = Insert Into Array(array=w1466, new element=w1404) -> (w1459:dbl[][])  [unwired: 2 in]
        n404 = Transpose 2D Array(2D array=w1459) -> (transposed array=w1458:dbl[][])
        n405 = call <vilib>:"compatOverwrite.vi"("overwrite (F)"=TRUE) -> ("overwrite?"=w1441:T8)
        n406 = Open/Create/Replace File(file path (use dialog)=w1464, error in=w1455, operation (0:open)=w1441) -> (refnum out=w1470:refnum<file>, error out=w1469:errorcluster)  [unwired: 3 in, 1 out]
        n407 = call "4155C Write array to file.vi"("Byte Stream File Refnum"=w1470, "Header"=string[] ["Time /s", "Ig /A", "Id /A", "Is /A"], "Data Array"=w1458, "error in (no error)"=w1469) -> ("dup refnum"=w1472:refnum<file>, "error out"=w1471:errorcluster)  [unwired: 1 in]
        n408 = Close File(refnum=w1472, error in=w1471) -> (error out=w1462:errorcluster)  [unwired: 1 out]
      }
      frame "samplei" {
        n409 = local read "Sample I - Source/Common"() -> (w1544:u32)
        n410 = Number To Decimal String(number=w1569) -> (decimal integer string=w1620:string)  [unwired: 1 in]
        n411 = local read "Sample I - Probe 4 (Disabled)"() -> (w1547:u32)
        n412 = Concatenate Strings(w1599, "-samplei-" ("Substring"), w1620, w1568, ".txt" ("Substring")) -> (w1618:string)
        n413 = Fract/Exp String To Number(string=w1617) -> (number=w1584:dbl[])  [unwired: 3 in, 1 out]
        n414 = String To Path(string=w1618) -> (path=w1602:path)
        n415 = local read "Sample I - Probe 3 (Disabled)"() -> (w1546:u32)
        n416 = Index Array(array=w1584, index=4 ("Index")) -> (element=w1578:dbl)
        n417 = Index Array(array=w1584, index=3 ("Index")) -> (element=w1579:dbl)
        n418 = Index Array(array=w1584, index=1 ("Index")) -> (element=w1581:dbl)
        n419 = Index Array(array=w1584, index=0 ("Index")) -> (element=w1582:dbl)
        n420 = Index Array(array=w1584, index=2 ("Index")) -> (element=w1580:dbl)
        n421 = local read "Sample I - Drain/Gate"() -> (w1545:u32)
        n422 = call "4155C Config SamplingI Measurements v2.0.vi"("VISA session"=w1623, "Num Points"=w1581, "Sample I - Probe 3 (Disabled)"=w1546, "Display on/off"=TRUE, "Sample I - Source/Common"=w1544, "Sample I - Drain/Gate"=w1545, "Sampling interval"=w1579, "Standby"=w1548, "error in (no error)"=w1622, "Timings"=w1591, "Sample I - Probe 4 (Disabled)"=w1547, "Sample time"=w1580) -> ("dup VISA resource name"=w1625:refnum<visa-resource-name>, "error out"=w1624:errorcluster)  [unwired: 2 in]
        n423 = call "4155C Take SampleI v2.0.vi"("Sample I - Drain/Gate"=w1545, "Emergency Stop"=w1596, "error in (no error)"=w1624, "Idg 2"=w1582, "Vdg compliance 2"=w1578, "VISA resource name in"=w1625) -> ("error out"=w1594:errorcluster, "Idg"=w1627:dbl[], "Vdg"=w1604:dbl[], "VISA Resource Name out"=w1592:refnum<visa-resource-name>, "Is"=w1626:dbl[], "Time"=w1608:dbl[])
        n424 = Insert Into Array(array=dbl[][] [] ("Input Array"), new element=w1608) -> (w1607:dbl[][])  [unwired: 2 in]
        n425 = Insert Into Array(array=w1607, new element=w1604) -> (w1606:dbl[][])  [unwired: 2 in]
        n426 = Insert Into Array(array=w1606, new element=w1627) -> (w1605:dbl[][])  [unwired: 2 in]
        n427 = VISA Write(VISA resource name=w1592, write buffer=":DISP ON" ("write buffer (\"\")"), error in (no error)=w1594) -> (VISA resource name out=w1577:refnum<visa-resource-name>, error out=w1593:errorcluster)  [unwired: 1 out]
        n428 = Insert Into Array(array=w1605, new element=w1626) -> (w1598:dbl[][])  [unwired: 2 in]
        n429 = call <vilib>:"compatOverwrite.vi"("overwrite (F)"=TRUE) -> ("overwrite?"=w1572:T8)
        n430 = Open/Create/Replace File(file path (use dialog)=w1602, error in=w1593, operation (0:open)=w1572) -> (refnum out=w1611:refnum<file>, error out=w1610:errorcluster)  [unwired: 3 in, 1 out]
        n431 = Transpose 2D Array(2D array=w1598) -> (transposed array=w1597:dbl[][])
        n432 = call "4155C Write array to file.vi"("Byte Stream File Refnum"=w1611, "Header"=string[] ["Time /s", "Vdg /V", "Idg /A", "Is /A"], "Data Array"=w1597, "error in (no error)"=w1610) -> ("dup refnum"=w1613:refnum<file>, "error out"=w1612:errorcluster)  [unwired: 1 in]
        n433 = Close File(refnum=w1613, error in=w1612) -> (error out=w1575:errorcluster)  [unwired: 1 out]
        n434 = VISA Write(VISA resource name=w1577, write buffer=";:PAGE:SCON:STAN OFF;:PAGE:CHAN:VSU2:DIS;" ("write buffer (\"\")"), error in (no error)=w1575) -> (VISA resource name out=w1573:refnum<visa-resource-name>, error out=w1574:errorcluster)  [unwired: 1 out]
      }
      frame "#" {
        n435 = VISA Write(VISA resource name=w1652, write buffer=":DISP ON" ("write buffer (\"\")"), error in (no error)=w1651) -> (VISA resource name out=w1650:refnum<visa-resource-name>, error out=w1649:errorcluster)  [unwired: 1 out]
      }
      frame "stressV" {
        n436 = Number To Decimal String(number=w1683) -> (decimal integer string=w1724:string)  [unwired: 1 in]
        n437 = Concatenate Strings(w1708, "-stressV-" ("Substring"), w1724, w1682, ".txt" ("Substring")) -> (w1722:string)
        n438 = Fract/Exp String To Number(string=w1721) -> (number=w1694:dbl[])  [unwired: 3 in, 1 out]
        n439 = local read "Stress V - Drain"() -> (w1661:u32)
        n440 = String To Path(string=w1722) -> (path=w1712:path)
        n441 = Index Array(array=w1694, index=3 ("Index")) -> (element=w1691:dbl)
        n442 = Index Array(array=w1694, index=1 ("Index")) -> (element=w1689:dbl)
        n443 = Index Array(array=w1694, index=0 ("Index")) -> (element=w1688:dbl)
        n444 = Index Array(array=w1694, index=4 ("Index")) -> (element=w1693:dbl)
        n445 = Index Array(array=w1694, index=2 ("Index")) -> (element=w1690:dbl)
        n446 = local read "Stress V - Gate"() -> (w1662:u32)
        n447 = local read "Stress V - Source/Common"() -> (w1663:u32)
        n448 = call "4155C Config V Stress v2.0.vi"("Display on/off"=TRUE, "Stress V - Gate"=w1662, "Stress V - Drain"=w1661, "Stress V - Source/Common"=w1663, "IG compliance"=w1690, "ID compliance"=w1691, "error in (no error)"=w1726, "VG"=w1688, "VD"=w1689, "VISA session"=w1727) -> ("error out"=w1728:errorcluster, "dup VISA resource name"=w1729:refnum<visa-resource-name>)
        n449 = call "4155C Apply Stress.vi"("error in (no error)"=w1728, "Duration"=w1693, "Emergency Stop"=w1707, "VISA resource name in"=w1729) -> ("error out"=w1705:errorcluster, "VISA Resource Name out"=w1703:refnum<visa-resource-name>)
        n450 = VISA Write(VISA resource name=w1703, write buffer=":DISP ON" ("write buffer (\"\")"), error in (no error)=w1705) -> (VISA resource name out=w1702:refnum<visa-resource-name>, error out=w1704:errorcluster)  [unwired: 1 out]
        n451 = call <vilib>:"compatOverwrite.vi"("overwrite (F)"=TRUE) -> ("overwrite?"=w1687:T8)
        n452 = Open/Create/Replace File(file path (use dialog)=w1712, error in=w1704, operation (0:open)=w1687) -> (refnum out=w1715:refnum<file>, error out=w1714:errorcluster)  [unwired: 3 in, 1 out]
        n453 = call "4155C Write array to file.vi"("Byte Stream File Refnum"=w1715, "Header"=string[] ["V stress completed successfully", ""], "error in (no error)"=w1714) -> ("dup refnum"=w1717:refnum<file>, "error out"=w1716:errorcluster)  [unwired: 2 in]
        n454 = Close File(refnum=w1717, error in=w1716) -> (error out=w1710:errorcluster)  [unwired: 1 out]
      }
      frame "stressI" {
        n455 = Number To Decimal String(number=w1751) -> (decimal integer string=w1788:string)  [unwired: 1 in]
        n456 = Concatenate Strings(w1772, "-stressI-" ("Substring"), w1788, w1750, ".txt" ("Substring")) -> (w1786:string)
        n457 = Fract/Exp String To Number(string=w1785) -> (number=w1760:dbl[])  [unwired: 3 in, 1 out]
        n458 = local read "Stress I - Source/Common"() -> (w1730:u32)
        n459 = Index Array(array=w1760, index=1 ("Index")) -> (element=w1756:dbl)
        n460 = Index Array(array=w1760, index=0 ("Index")) -> (element=w1757:dbl)
        n461 = Index Array(array=w1760, index=2 ("Index")) -> (element=w1758:dbl)
        n462 = String To Path(string=w1786) -> (path=w1776:path)
        n463 = local read "Stress I - Drain/Gate"() -> (w1731:u32)
        n464 = call "4155C Config I Stress v2.0.vi"("Stress I - Drain/Gate"=w1731, "Stress I - Source/Common"=w1730, "Display on/off"=TRUE, "error in (no error)"=w1790, "VDG compliance"=w1756, "IDG"=w1757, "VISA session"=w1791) -> ("error out"=w1792:errorcluster, "dup VISA resource name"=w1793:refnum<visa-resource-name>)  [unwired: 1 in]
        n465 = call "4155C Apply Stress.vi"("error in (no error)"=w1792, "Duration"=w1758, "Emergency Stop"=w1771, "VISA resource name in"=w1793) -> ("error out"=w1769:errorcluster, "VISA Resource Name out"=w1767:refnum<visa-resource-name>)
        n466 = VISA Write(VISA resource name=w1767, write buffer=":DISP ON" ("write buffer (\"\")"), error in (no error)=w1769) -> (VISA resource name out=w1766:refnum<visa-resource-name>, error out=w1768:errorcluster)  [unwired: 1 out]
        n467 = call <vilib>:"compatOverwrite.vi"("overwrite (F)"=TRUE) -> ("overwrite?"=w1755:T8)
        n468 = Open/Create/Replace File(file path (use dialog)=w1776, error in=w1768, operation (0:open)=w1755) -> (refnum out=w1779:refnum<file>, error out=w1778:errorcluster)  [unwired: 3 in, 1 out]
        n469 = call "4155C Write array to file.vi"("Byte Stream File Refnum"=w1779, "Header"=string[] ["I stress completed successfully", ""], "error in (no error)"=w1778) -> ("dup refnum"=w1781:refnum<file>, "error out"=w1780:errorcluster)  [unwired: 2 in]
        n470 = Close File(refnum=w1781, error in=w1780) -> (error out=w1774:errorcluster)  [unwired: 1 out]
      }
      frame "vsu2pulse" {
        n471 = Number To Decimal String(number=w1814) -> (decimal integer string=w1849:string)  [unwired: 1 in]
        n472 = Concatenate Strings(w1834, "-vsu2-" ("Substring"), w1849, w1813, ".txt" ("Substring")) -> (w1847:string)
        n473 = Fract/Exp String To Number(string=w1846) -> (number=w1822:dbl[])  [unwired: 3 in, 1 out]
        n474 = String To Path(string=w1847) -> (path=w1838:path)
        n475 = Index Array(array=w1822, index=1 ("Index")) -> (element=w1821:dbl)
        n476 = Index Array(array=w1822, index=0 ("Index")) -> (element=w1819:dbl)
        n477 = local read "VSU2 Stress - Source/Common"() -> (w1794:u32)
        n478 = call "4155C Config VSU2 Stress v2.0.vi"("VISA session"=w1852, "Display on/off"=TRUE, "VSU2"=w1819, "error in (no error)"=w1851, "VSU2 Stress - Source/Common"=w1794) -> ("dup VISA resource name"=w1854:refnum<visa-resource-name>, "error out"=w1853:errorcluster)
        n479 = call "4155C Apply Stress.vi"("error in (no error)"=w1853, "Duration"=w1821, "Emergency Stop"=w1833, "VISA resource name in"=w1854) -> ("error out"=w1831:errorcluster, "VISA Resource Name out"=w1829:refnum<visa-resource-name>)
        n480 = VISA Write(VISA resource name=w1829, write buffer=":DISP ON" ("write buffer (\"\")"), error in (no error)=w1831) -> (VISA resource name out=w1828:refnum<visa-resource-name>, error out=w1830:errorcluster)  [unwired: 1 out]
        n481 = call <vilib>:"compatOverwrite.vi"("overwrite (F)"=TRUE) -> ("overwrite?"=w1818:T8)
        n482 = Open/Create/Replace File(file path (use dialog)=w1838, error in=w1830, operation (0:open)=w1818) -> (refnum out=w1841:refnum<file>, error out=w1840:errorcluster)  [unwired: 3 in, 1 out]
        n483 = call "4155C Write array to file.vi"("Byte Stream File Refnum"=w1841, "Header"=string[] ["VSU2 pulse completed successfully", ""], "error in (no error)"=w1840) -> ("dup refnum"=w1843:refnum<file>, "error out"=w1842:errorcluster)  [unwired: 2 in]
        n484 = Close File(refnum=w1843, error in=w1842) -> (error out=w1836:errorcluster)  [unwired: 1 out]
      }
      frame "sample-fpp" {
        w1890 = string[] ["Time /s", "Id VgVd /A", "Ig VgVd /A", "Vp1 VgVd /V", "Vp2 VgVd /V"] ("Header")
        w1894 = "%d" ("format string")
        n485 = local read "FPP - Drain"() -> (w1856:u32)
        n486 = local read "FPP - Source"() -> (w1855:u32)
        n487 = Fract/Exp String To Number(string=w1939) -> (number=w1927:dbl[])  [unwired: 3 in, 1 out]
        n488 = local read "FPP - Probe 1"() -> (w1859:u32)
        n489 = Number To Decimal String(number=w1880) -> (decimal integer string=w1942:string)  [unwired: 1 in]
        n490 = Concatenate Strings(w1933, "-samplefpp-" ("Substring"), w1942, w1879, ".txt" ("Substring")) -> (w1940:string)
        n491 = local read "FPP - Gate"() -> (w1857:u32)
        n492 = String To Path(string=w1940) -> (path=w1902:path)
        n493 = local read "FPP - Probe 2"() -> (w1858:u32)
        n494 = Index Array(array=w1927, index=0 ("Index")) -> (element=w1889:dbl)
        n495 = Index Array(array=w1927, index=1 ("Index")) -> (element=w1888:dbl)
        n496 = Index Array(array=w1927, index=2 ("Index")) -> (element=w1935:dbl)
        n497 = Index Array(array=w1927, index=3 ("Index")) -> (element=w1925:dbl)
        n498 = call "4155C Config Sampling Measurements FPP v2.0.vi"("VISA session"=w1945, "Gate Compliance"=w1934, "FPP - Source"=w1855, "FPP - Drain"=w1856, "Drain Compliance"=w1943, "error in (no error)"=w1944, "Num Points"=w1935, "Timings"=w1932, "FPP - Gate"=w1857, "FPP - Probe 1"=w1859, "Vg"=w1889, "Vd"=w1888, "Display on/off"=TRUE, "Sample time"=w1925, "FPP - Probe 2"=w1858, "Standby"=w1860) -> ("dup VISA resource name"=w1904:refnum<visa-resource-name>, "error out"=w1903:errorcluster)  [unwired: 2 in]
        n499 = Number To Decimal String(number=w1889) -> (decimal integer string=w1914:string)  [unwired: 1 in]
        n500 = call "4155C Take Sample FPP.vi"("VISA resource name in"=w1904, "error in (no error)"=w1903, "Emergency Stop"=w1905) -> ("Time"=w1909:dbl[], "Vp1"=w1919:dbl[], "VISA Resource Name out"=w1886:refnum<visa-resource-name>, "Ig"=w1907:dbl[], "Id"=w1908:dbl[], "Vp2"=w1917:dbl[], "error out"=w1906:errorcluster)  [unwired: 10 in]
        n501 = Insert Into Array(array=dbl[][] [] ("Input Array"), new element=w1909) -> (w1923:dbl[][])  [unwired: 2 in]
        n502 = Number To Decimal String(number=w1888) -> (decimal integer string=w1912:string)  [unwired: 1 in]
        n503 = Insert Into Array(array=w1923, new element=w1908) -> (w1922:dbl[][])  [unwired: 2 in]
        n504 = Concatenate Strings("(Vg = " ("Substring"), w1914, "V, Vd = " ("Substring"), w1912, "V)" ("Substring")) -> (w1910:string)
        n505 = Insert Into Array(array=w1922, new element=w1907) -> (w1921:dbl[][])  [unwired: 2 in]
        n506 = Insert Into Array(array=w1921, new element=w1919) -> (w1918:dbl[][])  [unwired: 2 in]
        n507 = Insert Into Array(array=w1918, new element=w1917) -> (w1887:dbl[][])  [unwired: 2 in]
        n508 = Transpose 2D Array(2D array=w1887) -> (transposed array=w1916:dbl[][])
        n509 = call <vilib>:"compatOverwrite.vi"("overwrite (F)"=TRUE) -> ("overwrite?"=w1884:T8)
        n510 = Open/Create/Replace File(file path (use dialog)=w1902, error in=w1906, operation (0:open)=w1884) -> (refnum out=w1899:refnum<file>, error out=w1900:errorcluster)  [unwired: 3 in, 1 out]
        n511 = Array To Spreadsheet String(array=w1890, 3:w1894) -> (spreadsheet string=w1896:string)  [unwired: 1 in]
        n512 = Search and Replace String(replace all?=TRUE ("replace all? (F)"), input string=w1896, search string="VgVd", replace string=w1910) -> (result string=w1892:string)  [unwired: 4 in, 3 out]
        n513 = Spreadsheet String To Array(format string=w1894, spreadsheet string=w1892, array type (2D Dbl)=w1890) -> (array=w1891:string[])  [unwired: 1 in]
        n514 = call "4155C Write array to file.vi"("Byte Stream File Refnum"=w1899, "Header"=w1891, "Data Array"=w1916, "error in (no error)"=w1900) -> ("dup refnum"=w1897:refnum<file>, "error out"=w1898:errorcluster)  [unwired: 1 in]
        n515 = Close File(refnum=w1897, error in=w1898) -> (error out=w1885:errorcluster)  [unwired: 1 out]
      }
      frame "resample-fpp" {
        w1978 = string[] ["Time /s", "Id VgVd /A", "Ig VgVd /A", "Vp1 VgVd /V", "Vp2 VgVd /V"] ("Header")
        w1982 = "%d" ("format string")
        n516 = Number To Decimal String(number=w1964) -> (decimal integer string=w2022:string)  [unwired: 1 in]
        n517 = Fract/Exp String To Number(string=w2019) -> (number=w1971:dbl[])  [unwired: 3 in, 1 out]
        n518 = Concatenate Strings(w2015, "-resamplefpp-" ("Substring"), w2022, w1965, ".txt" ("Substring")) -> (w2020:string)
        n519 = String To Path(string=w2020) -> (path=w1990:path)
        n520 = Index Array(array=w1971, index=0 ("Index")) -> (element=w1977:dbl)
        n521 = Index Array(array=w1971, index=1 ("Index")) -> (element=w1976:dbl)
        n522 = Number To Decimal String(number=w1977) -> (decimal integer string=w2000:string)  [unwired: 1 in]
        n523 = call "4155C Take Sample FPP.vi"("VISA resource name in"=w1973, "error in (no error)"=w1972, "Emergency Stop"=w1991) -> ("Time"=w1995:dbl[], "Vp1"=w2005:dbl[], "VISA Resource Name out"=w1975:refnum<visa-resource-name>, "Ig"=w1993:dbl[], "Id"=w1994:dbl[], "Vp2"=w2003:dbl[], "error out"=w1992:errorcluster)  [unwired: 10 in]
        n524 = Insert Into Array(array=dbl[][] [] ("Input Array"), new element=w1995) -> (w2009:dbl[][])  [unwired: 2 in]
        n525 = Number To Decimal String(number=w1976) -> (decimal integer string=w1998:string)  [unwired: 1 in]
        n526 = Insert Into Array(array=w2009, new element=w1994) -> (w2008:dbl[][])  [unwired: 2 in]
        n527 = Concatenate Strings("(Vg = " ("Substring"), w2000, "V, Vd = " ("Substring"), w1998, "V)" ("Substring")) -> (w1996:string)
        n528 = Insert Into Array(array=w2008, new element=w1993) -> (w2007:dbl[][])  [unwired: 2 in]
        n529 = Insert Into Array(array=w2007, new element=w2005) -> (w2004:dbl[][])  [unwired: 2 in]
        n530 = Insert Into Array(array=w2004, new element=w2003) -> (w1970:dbl[][])  [unwired: 2 in]
        n531 = call <vilib>:"compatOverwrite.vi"("overwrite (F)"=TRUE) -> ("overwrite?"=w1969:T8)
        n532 = Open/Create/Replace File(file path (use dialog)=w1990, error in=w1992, operation (0:open)=w1969) -> (refnum out=w1987:refnum<file>, error out=w1988:errorcluster)  [unwired: 3 in, 1 out]
        n533 = Array To Spreadsheet String(array=w1978, 3:w1982) -> (spreadsheet string=w1984:string)  [unwired: 1 in]
        n534 = Transpose 2D Array(2D array=w1970) -> (transposed array=w2002:dbl[][])
        n535 = Search and Replace String(replace all?=TRUE ("replace all? (F)"), input string=w1984, search string="VgVd", replace string=w1996) -> (result string=w1980:string)  [unwired: 4 in, 3 out]
        n536 = Spreadsheet String To Array(format string=w1982, spreadsheet string=w1980, array type (2D Dbl)=w1978) -> (array=w1979:string[])  [unwired: 1 in]
        n537 = call "4155C Write array to file.vi"("Byte Stream File Refnum"=w1987, "Header"=w1979, "Data Array"=w2002, "error in (no error)"=w1988) -> ("dup refnum"=w1985:refnum<file>, "error out"=w1986:errorcluster)  [unwired: 1 in]
        n538 = Close File(refnum=w1985, error in=w1986) -> (error out=w1974:errorcluster)  [unwired: 1 out]
      }
      frame "serial" {
        n539 = local read "Termination char\n(0xA = '\\n' = LF)\n(0xD = '\\r' = CR)"() -> (w2049:u8)
        n540 = local read "Enable Termination\nChar (T)"() -> (w2050:bool)
        n541 = Index Array(array=w2057, index=0 ("Index")) -> (element=w2056:string)
        n542 = local read "parity"() -> (w2040:u16)
        n543 = local read "Delay before read (ms)"() -> (w2051:u32)
        n544 = local read "byte count"() -> (w2048:u32)
        n545 = local read "Timeout (ms)"() -> (w2047:u32)
        n546 = local read "VISA resource name"() -> (w2044:refnum<visa-resource-name>)
        n547 = local read "baud rate"() -> (w2043:u32)
        n548 = local read "Serial End Mode for Reads"() -> (w2042:u16)
        n549 = local read "data bits"() -> (w2041:u16)
        n550 = local read "stop bits"() -> (w2046:u16)
        n551 = local read "flow control"() -> (w2045:u16)
        n552 = call "Serial write and read v0.5.vi"("Delay before read (ms)"=w2051, "Termination char\n(0xA = '\\n' = LF)\n(0xD = '\\r' = CR)"=w2049, "Enable Termination\nChar (T)"=w2050, "parity"=w2040, "stop bits"=w2046, "string to write"=w2056, "flow control"=w2045, "byte count"=w2048, "Serial Settings:Serial End Mode for Reads"=w2042, "Timeout (ms)"=w2047, "error in (no error)"=w2062, "VISA resource name"=w2044, "baud rate"=w2043, "data bits"=w2041) -> ("Serial port output"=w2052:string, "error out"=w2061:errorcluster)
        n553 = Build Array (concatenate)(w2052, w2053) -> (w2054:string[])
      }
    }
    n554 = local read "Time Units"() -> (w97:u16)
    n555 = case shown="0" w97 {
      tunnel: ["Time (Seconds)" ("element") "Time (Minutes)" ("element") "Time (Hours)" ("element")] -> w135
      frame 0 {
      }
      frame 1, Default {
      }
      frame 2 {
      }
    }
    n556 = Build Array(w147, w103, w113, w112, w111, w110, w109, w108, w107, w106, w105, w104, w102) -> (w168:dbl[][])
    n557 = Transpose 2D Array(2D array=w168) -> (transposed array=w167:dbl[][])
    n558 = Concatenate Strings(w69, "-Imax_Imin_Ion_Ioff_vs_time.txt" ("Suffix (Imax,Imin,Ion,Ioff)")) -> (w178:string)
    n559 = Build Array(w135, "Is max (A)" ("VAR2 Name"), "Is min (A)" ("VAR2 Name"), "Id max (A)" ("VAR2 Name"), "Id min (A)" ("VAR2 Name"), "Ig max (A)" ("VAR2 Name"), "Ig min (A)" ("VAR2 Name"), "Is on (A)" ("VAR2 Name"), "Is off (A)" ("VAR2 Name"), "Id on (A)" ("VAR2 Name"), "Id off (A)" ("VAR2 Name"), "Ig on (A)" ("VAR2 Name"), "Ig off (A)" ("VAR2 Name")) -> (w173:string[])
    n560 = Array To Spreadsheet String(array=w167, 3:"%e" ("format string")) -> (spreadsheet string=w171:string)  [unwired: 1 in]
    n561 = Array To Spreadsheet String(array=w173, 3:"" ("format string")) -> (spreadsheet string=w172:string)  [unwired: 1 in]
    n562 = String To Path(string=w178) -> (path=w177:path)
    n563 = Build Array(w172, w171) -> (w170:string[])
    n564 = Write to Text File(file (use dialog)=w177, text=w170, error in=w146) -> (refnum out=w179:refnum<file>, error out=w169:errorcluster)  [unwired: 1 in, 1 out]
    n565 = Close File(refnum=w179, error in=w169) -> (error out=w100:errorcluster)  [unwired: 1 out]
    n566 = Concatenate Strings(w69, "-serial_port_output.txt" ("Suffix (serial port log)")) -> (w149:string)
    n567 = String To Path(string=w149) -> (path=w148:path)
    n568 = Build Array(w135, "Serial port input" ("VAR2 Name"), "Serial port output: ") -> (w139:string[])
    n569 = Array To Spreadsheet String(array=w143, 3:"" ("format string")) -> (spreadsheet string=w136:string)  [unwired: 1 in]
    n570 = Array To Spreadsheet String(array=w139, 3:"" ("format string")) -> (spreadsheet string=w137:string)  [unwired: 1 in]
    n571 = Build Array(w137, w136) -> (w138:string[])
    n572 = Array To Spreadsheet String(array=w142, 3:"" ("format string")) -> (spreadsheet string=w154:string)  [unwired: 1 in]
    n573 = Write to Text File(file (use dialog)=w148, text=w138, error in=w100) -> (refnum out=w150:refnum<file>, error out=w151:errorcluster)  [unwired: 1 in, 1 out]
    n574 = Close File(refnum=w150, error in=w151) -> (error out=w71:errorcluster)  [unwired: 1 out]
    n575 = local write "Serial port data"(w154) -> ()
    n576 = Build Array(w68, w67, w66, w65) -> (w81:dbl[][])
    n577 = Build Array("Time (Seconds)" ("element"), "Is (A)" ("VAR2 Name"), "Id (A)" ("VAR2 Name"), "Ig (A)" ("VAR2 Name")) -> (w77:string[])
    n578 = Transpose 2D Array(2D array=w81) -> (transposed array=w80:dbl[][])
    n579 = Concatenate Strings(w69, "-sample_vs_time.txt" ("Suffix (Imax,Imin,Ion,Ioff)")) -> (w87:string)
    n580 = Array To Spreadsheet String(array=w77, 3:"" ("format string")) -> (spreadsheet string=w76:string)  [unwired: 1 in]
    n581 = Array To Spreadsheet String(array=w80, 3:"%e" ("format string")) -> (spreadsheet string=w84:string)  [unwired: 1 in]
    n582 = String To Path(string=w87) -> (path=w86:path)
    n583 = Build Array(w76, w84) -> (w83:string[])
    n584 = Write to Text File(file (use dialog)=w86, text=w83, error in=w71) -> (refnum out=w88:refnum<file>, error out=w82:errorcluster)  [unwired: 1 in, 1 out]
    n585 = Close File(refnum=w88, error in=w82) -> (error out=w70:errorcluster)  [unwired: 1 out]
  }
  "error out" <- w27
  "Timings Indicator" <- w19
  "Probe 4 Indicator" <- w3
  "Is max" <- w13
  "Id max" <- w13
  "Ig max" <- w13
  "Imax vs time" <- w2
  "I vs Vg" <- w2
  "Imin vs time" <- w2
  "I vs Vd" <- w2
  "Serial port data" <- "" ("Serial port data")
  "Is min" <- w12
  "Id min" <- w12
  "Ig min" <- w12
  "Ion vs time" <- w2
  "Ioff vs time" <- w2
  "Is on" <- w11
  "Id on" <- w11
  "Ig on" <- w11
  "Is off" <- w10
  "Id off" <- w10
  "Ig off" <- w10
  "I vs time (Bias Stress)" <- w2
